vi "main_Extended-Kalman Filter.vi"() -> ()   [LabVIEW 2019]
uses:
  <vilib>/Analysis/Matrix/Datatypes/RealMatrix.ctl
  Ctrl/cmd_common.ctl
  Ctrl/cmd_ini-RW.ctl
  <vilib>/Analysis/Matrix/NI_Matrix.lvlib
panel:
  in  "tab":enum32{"ini val", "Graph"}(tab)=enum."Graph"
  out "GNSS Lat-Long":T1(graph)=[{[{"Real Matrix Element"=0.00648229933015812, "Real Matrix Element"=-0.1485998715838205}, {"Real Matrix Element"=0.13764030324676432, "Real Matrix Element"=-0.031872708572077454}, {"Real Matrix Element"=0.2814176053656353, "Real Matrix Element"=-0.18668844986322813}, {"Real Matrix Element"=0.4677656590914504, "Real Matrix Element"=-0.0031668042546943997}, {"Real Matrix Element"=0.4503900731423714, "Real Matrix Element"=-0.03691015780949122}, {"Real Matrix Element"=0.49534101114982676, "Real Matrix Element"=-0.0424373953622008}, {"Real Matrix Element"=0.5298272405394908, "Real Matrix Element"=-0.018737920527740447}, {"Real Matrix Element"=0.6136709918692839, "Real Matrix Element"=-0.07905311271886954}, {"Real Matrix Element"=0.8672293050090724, "Real Matrix Element"=0.11930935270810816}, {"Real Matrix Element"=1.032724976114411, "Real Matrix Element"=-0.028094767288573047}, {"Real Matrix Element"=1.025639298375923, "Real Matrix Element"=-0.015205341516983151}, {"Real Matrix Element"=1.0403214942691346, "Real Matrix Element"=0.10295017559703463}, {"Real Matrix Element"=1.2192703763694923, "Real Matrix Element"=0.2632396677335336}, {"Real Matrix Element"=1.2484932187390043, "Real Matrix Element"=0.11930141709508046}, {"Real Matrix Element"=1.28679874101843, "Real Matrix Element"=0.3188853450127311}, {"Real Matrix Element"=1.2528049501602503, "Real Matrix Element"=0.20840561524288012}, {"Real Matrix Element"=1.5260015333317185, "Real Matrix Element"=0.20710760450243698}, {"Real Matrix Element"=1.5664918211546404, "Real Matrix Element"=0.13271924379662997}, {"Real Matrix Element"=1.8460444096776403, "Real Matrix Element"=0.2388525674226506}, {"Real Matrix Element"=1.7893086393547315, "Real Matrix Element"=0.23473315440221695}, {"Real Matrix Element"=2.1003619347831006, "Real Matrix Element"=0.18965751247444596}, {"Real Matrix Element"=2.1527235912017235, "Real Matrix Element"=0.21292351546767185}, {"Real Matrix Element"=2.0471398164787855, "Real Matrix Element"=0.24502152593798443}, {"Real Matrix Element"=2.246363828219961, "Real Matrix Element"=0.21555940024166098}, {"Real Matrix Element"=2.3610927477240558, "Real Matrix Element"=0.2478574057445659}, {"Real Matrix Element"=2.4439556028948055, "Real Matrix Element"=0.34991078944230897}, {"Real Matrix Element"=2.4855190346914235, "Real Matrix Element"=0.4958049830178777}, {"Real Matrix Element"=2.677137946482532, "Real Matrix Element"=0.415459813566203}, {"Real Matrix Element"=2.8400473959196373, "Real Matrix Element"=0.3729959888015044}, {"Real Matrix Element"=2.8126782352199013, "Real Matrix Element"=0.3900898497303645}, {"Real Matrix Element"=3.0316200287530095, "Real Matrix Element"=0.41711101629898045}, {"Real Matrix Element"=3.159342773172584, "Real Matrix Element"=0.48895603096833595}, {"Real Matrix Element"=3.1177640465501595, "Real Matrix Element"=0.5990497173429132}, {"Real Matrix Element"=3.431510484521816, "Real Matrix Element"=0.6923490256189043}, {"Real Matrix Element"=3.6265865881623625, "Real Matrix Element"=0.7358839573835992}, {"Real Matrix Element"=3.678232807948232, "Real Matrix Element"=0.68180069643571}, {"Real Matrix Element"=3.765659578050578, "Real Matrix Element"=0.8018945377182328}, {"Real Matrix Element"=3.6248552222086228, "Real Matrix Element"=0.4741738414926855}, {"Real Matrix Element"=3.7222020295046874, "Real Matrix Element"=0.518341799011495}, {"Real Matrix Element"=3.9502494355664957, "Real Matrix Element"=0.7844506067834873}, {"Real Matrix Element"=4.140443942092801, "Real Matrix Element"=0.6861077494054908}, {"Real Matrix Element"=4.329408585769923, "Real Matrix Element"=0.9587932783737416}, {"Real Matrix Element"=4.4518189256360055, "Real Matrix Element"=0.9438312142162951}, {"Real Matrix Element"=4.565733385367433, "Real Matrix Element"=0.9829122817561525}, {"Real Matrix Element"=4.6100291786353536, "Real Matrix Element"=1.0160060370690478}, {"Real Matrix Element"=4.682015899254993, "Real Matrix Element"=1.1774809714765537}, {"Real Matrix Element"=4.732474262362473, "Real Matrix Element"=1.2571329943283698}, {"Real Matrix Element"=4.6216704645451285, "Real Matrix Element"=0.7679884807807758}, {"Real Matrix Element"=4.794245939393425, "Real Matrix Element"=0.7679902776857672}, {"Real Matrix Element"=4.856828698615568, "Real Matrix Element"=0.8294593794196793}, {"Real Matrix Element"=5.006091376727372, "Real Matrix Element"=0.9850119127052693}, {"Real Matrix Element"=5.173313411136047, "Real Matrix Element"=1.291609237984442}, {"Real Matrix Element"=5.196884811093232, "Real Matrix Element"=1.438539845070721}, {"Real Matrix Element"=5.269297502943308, "Real Matrix Element"=1.3591797613509908}, {"Real Matrix Element"=5.326632454975217, "Real Matrix Element"=1.5019081952917732}, {"Real Matrix Element"=5.53950476112955, "Real Matrix Element"=1.5954667192482002}, {"Real Matrix Element"=5.546075834353704, "Real Matrix Element"=1.5963373800411635}, {"Real Matrix Element"=5.50787264268229, "Real Matrix Element"=1.5136014331108896}, {"Real Matrix Element"=5.597318829657093, "Real Matrix Element"=1.6911722909521052}, {"Real Matrix Element"=5.745469013544655, "Real Matrix Element"=1.9741214083072083}, {"Real Matrix Element"=5.826534676656871, "Real Matrix Element"=1.8362557577429413}, {"Real Matrix Element"=5.777420682360288, "Real Matrix Element"=1.6471604684917265}, {"Real Matrix Element"=5.783642698159415, "Real Matrix Element"=1.7983117212024493}, {"Real Matrix Element"=5.77706746416779, "Real Matrix Element"=1.5876776162294384}, {"Real Matrix Element"=6.070669468161333, "Real Matrix Element"=2.0406137236959054}, {"Real Matrix Element"=6.1820279880490645, "Real Matrix Element"=2.043202141200636}, {"Real Matrix Element"=6.219822211005529, "Real Matrix Element"=2.099773718842126}, {"Real Matrix Element"=6.295561619993403, "Real Matrix Element"=1.9409629598593416}, {"Real Matrix Element"=6.439200544048959, "Real Matrix Element"=2.0875731372661637}, {"Real Matrix Element"=6.457028372016953, "Real Matrix Element"=2.203865379008531}, {"Real Matrix Element"=6.4704852502079975, "Real Matrix Element"=2.6003188639731913}, {"Real Matrix Element"=6.554666254302385, "Real Matrix Element"=2.503194424454099}, {"Real Matrix Element"=6.5733554844620565, "Real Matrix Element"=2.480092898008009}, {"Real Matrix Element"=6.754152844278384, "Real Matrix Element"=2.728791386153097}, {"Real Matrix Element"=6.674564513462208, "Real Matrix Element"=2.300939933732716}, {"Real Matrix Element"=6.691289619645367, "Real Matrix Element"=2.559983090203076}, {"Real Matrix Element"=6.8947220042735005, "Real Matrix Element"=2.7230740025712734}, {"Real Matrix Element"=7.015805006692874, "Real Matrix Element"=2.9921120011808027}, {"Real Matrix Element"=7.134483557016957, "Real Matrix Element"=2.887264461377884}, {"Real Matrix Element"=7.102799773965878, "Real Matrix Element"=2.863049574205883}, {"Real Matrix Element"=7.096532109525193, "Real Matrix Element"=3.000878596933252}, {"Real Matrix Element"=7.278203294615071, "Real Matrix Element"=3.2591886274505706}, {"Real Matrix Element"=7.267274013305502, "Real Matrix Element"=3.239806978191403}, {"Real Matrix Element"=7.432382425022456, "Real Matrix Element"=3.5891598453443536}, {"Real Matrix Element"=7.412170502397272, "Real Matrix Element"=3.4593252300230164}, {"Real Matrix Element"=7.535515352097216, "Real Matrix Element"=3.550645213044657}, {"Real Matrix Element"=7.735555416947001, "Real Matrix Element"=3.6444852552704137}, {"Real Matrix Element"=7.792479661433866, "Real Matrix Element"=3.5591098996316397}, {"Real Matrix Element"=7.932826704204354, "Real Matrix Element"=3.895277482405934}, {"Real Matrix Element"=7.873200422033903, "Real Matrix Element"=3.643453113387131}, {"Real Matrix Element"=7.9872990985151935, "Real Matrix Element"=3.7482458583440232}, {"Real Matrix Element"=8.023783453842626, "Real Matrix Element"=3.908963545529375}, {"Real Matrix Element"=8.090971345781176, "Real Matrix Element"=4.158683909791595}, {"Real Matrix Element"=8.179024885407793, "Real Matrix Element"=4.396388435221577}, {"Real Matrix Element"=8.244443630526025, "Real Matrix Element"=4.5010787950401925}, {"Real Matrix Element"=8.175467225219704, "Real Matrix Element"=4.304323569685333}, {"Real Matrix Element"=8.192177808998313, "Real Matrix Element"=4.296358269859259}, {"Real Matrix Element"=8.264968809143058, "Real Matrix Element"=4.25581006734387}, {"Real Matrix Element"=8.36355332414695, "Real Matrix Element"=4.410547430378274}, {"Real Matrix Element"=8.418999830088936, "Real Matrix Element"=4.441577526445436}, {"Real Matrix Element"=8.562267588591794, "Real Matrix Element"=4.527930122835036}, {"Real Matrix Element"=8.520294036398598, "Real Matrix Element"=4.864102834164672}, {"Real Matrix Element"=8.636696088427488, "Real Matrix Element"=4.9782078037972}, {"Real Matrix Element"=8.713850366189384, "Real Matrix Element"=4.962690664747354}, {"Real Matrix Element"=8.764321844517646, "Real Matrix Element"=5.114081495990158}, {"Real Matrix Element"=8.847549669446503, "Real Matrix Element"=5.218346627649721}, {"Real Matrix Element"=8.827369626773182, "Real Matrix Element"=5.021489079132804}, {"Real Matrix Element"=8.903059713218287, "Real Matrix Element"=5.235767123116211}, {"Real Matrix Element"=8.963155178977614, "Real Matrix Element"=5.598077779344656}, {"Real Matrix Element"=8.987948084499166, "Real Matrix Element"=5.597411139757482}, {"Real Matrix Element"=8.968808580972492, "Real Matrix Element"=5.645722006826326}, {"Real Matrix Element"=9.113001823113587, "Real Matrix Element"=5.60411213366905}, {"Real Matrix Element"=9.173522281833215, "Real Matrix Element"=5.852524519544907}, {"Real Matrix Element"=9.17913802407535, "Real Matrix Element"=6.032383124796971}, {"Real Matrix Element"=9.232914231961534, "Real Matrix Element"=5.837227051561382}, {"Real Matrix Element"=9.32071271816769, "Real Matrix Element"=6.001382731775994}, {"Real Matrix Element"=9.432490446545314, "Real Matrix Element"=6.077384745280501}, {"Real Matrix Element"=9.599670577348716, "Real Matrix Element"=6.3096112031527944}, {"Real Matrix Element"=9.671538974157912, "Real Matrix Element"=6.273083960801199}, {"Real Matrix Element"=9.577958664052026, "Real Matrix Element"=6.2972763478809926}, {"Real Matrix Element"=9.62603714326331, "Real Matrix Element"=6.374956836079589}, {"Real Matrix Element"=9.835344466832757, "Real Matrix Element"=6.4637793043762946}, {"Real Matrix Element"=9.909203846785434, "Real Matrix Element"=6.872950958027769}, {"Real Matrix Element"=9.840759582646996, "Real Matrix Element"=6.722130787954949}, {"Real Matrix Element"=9.973720776756435, "Real Matrix Element"=6.985178872427905}, {"Real Matrix Element"=9.945020881597433, "Real Matrix Element"=7.0799896615141265}, {"Real Matrix Element"=10.019541195927266, "Real Matrix Element"=6.961037799237819}, {"Real Matrix Element"=10.029458760055693, "Real Matrix Element"=6.770951391743203}, {"Real Matrix Element"=9.95680039378121, "Real Matrix Element"=6.894932057458966}, {"Real Matrix Element"=9.972679986203673, "Real Matrix Element"=7.097027209828476}, {"Real Matrix Element"=10.068459547490654, "Real Matrix Element"=7.346327751875404}, {"Real Matrix Element"=10.151213352812169, "Real Matrix Element"=7.3336762919149505}, {"Real Matrix Element"=10.090891521075756, "Real Matrix Element"=7.530166753288197}, {"Real Matrix Element"=10.147224053917913, "Real Matrix Element"=7.8719545623908855}, {"Real Matrix Element"=10.247445130984264, "Real Matrix Element"=8.059616854073887}, {"Real Matrix Element"=10.29353595886074, "Real Matrix Element"=7.9879086674452715}, {"Real Matrix Element"=10.226581274584332, "Real Matrix Element"=8.14872711101871}, {"Real Matrix Element"=10.182657003096221, "Real Matrix Element"=7.979886222894717}, {"Real Matrix Element"=10.170170736983122, "Real Matrix Element"=8.210361178998122}, {"Real Matrix Element"=10.221301770259442, "Real Matrix Element"=8.19710414327885}, {"Real Matrix Element"=10.23122536653524, "Real Matrix Element"=8.41557432626885}, {"Real Matrix Element"=10.22909019102822, "Real Matrix Element"=8.295293137067564}, {"Real Matrix Element"=10.36739039274229, "Real Matrix Element"=8.445827694791747}, {"Real Matrix Element"=10.39450178371217, "Real Matrix Element"=8.704741369116837}, {"Real Matrix Element"=10.568638625081983, "Real Matrix Element"=8.846568127767178}, {"Real Matrix Element"=10.559977944425762, "Real Matrix Element"=8.876524284264356}, {"Real Matrix Element"=10.696128835374578, "Real Matrix Element"=8.909886242456711}, {"Real Matrix Element"=10.68613966102341, "Real Matrix Element"=9.225666737988437}, {"Real Matrix Element"=10.638910101463535, "Real Matrix Element"=9.200847051506699}, {"Real Matrix Element"=10.641981226688847, "Real Matrix Element"=9.228452429971046}, {"Real Matrix Element"=10.65517617340279, "Real Matrix Element"=9.220194949369594}, {"Real Matrix Element"=10.691934312144625, "Real Matrix Element"=9.220574387761589}, {"Real Matrix Element"=10.856493342491829, "Real Matrix Element"=9.456143755756003}, {"Real Matrix Element"=10.748481161304678, "Real Matrix Element"=9.660792312776644}, {"Real Matrix Element"=10.730109086692375, "Real Matrix Element"=9.661757950863059}, {"Real Matrix Element"=10.71249938490896, "Real Matrix Element"=9.88205892199337}, {"Real Matrix Element"=10.519708404690254, "Real Matrix Element"=9.633758525080326}, {"Real Matrix Element"=10.537028139820096, "Real Matrix Element"=9.711517025179154}, {"Real Matrix Element"=10.611910728524084, "Real Matrix Element"=9.846185660821696}, {"Real Matrix Element"=10.651966971953641, "Real Matrix Element"=9.956538412771572}, {"Real Matrix Element"=10.716055814283216, "Real Matrix Element"=10.181348255220488}, {"Real Matrix Element"=10.738690953168351, "Real Matrix Element"=10.195158981215268}, {"Real Matrix Element"=10.81569244536906, "Real Matrix Element"=10.333686183942001}, {"Real Matrix Element"=10.891289126354476, "Real Matrix Element"=10.647008375840068}, {"Real Matrix Element"=10.945229634349461, "Real Matrix Element"=10.356736595320573}, {"Real Matrix Element"=11.036714501214382, "Real Matrix Element"=10.433679401177264}, {"Real Matrix Element"=11.095978460860579, "Real Matrix Element"=10.834554613260545}, {"Real Matrix Element"=10.962880721495313, "Real Matrix Element"=10.721611576289368}, {"Real Matrix Element"=10.945970437104213, "Real Matrix Element"=10.777251776751498}, {"Real Matrix Element"=10.858418050644882, "Real Matrix Element"=11.106073137748869}, {"Real Matrix Element"=10.992624941935272, "Real Matrix Element"=11.486243688704834}, {"Real Matrix Element"=10.738788257878593, "Real Matrix Element"=10.956412747643766}, {"Real Matrix Element"=10.883062812427877, "Real Matrix Element"=11.020596690664222}, {"Real Matrix Element"=11.107212545404389, "Real Matrix Element"=11.425304671954585}, {"Real Matrix Element"=11.067696675081926, "Real Matrix Element"=11.512956937565612}, {"Real Matrix Element"=11.160753482337359, "Real Matrix Element"=11.55748715945855}, {"Real Matrix Element"=11.073554637302253, "Real Matrix Element"=11.763495460705855}, {"Real Matrix Element"=11.138923802464973, "Real Matrix Element"=11.984706913691065}, {"Real Matrix Element"=11.155131070521213, "Real Matrix Element"=12.000895635212945}, {"Real Matrix Element"=11.156829831662023, "Real Matrix Element"=11.91719637666095}, {"Real Matrix Element"=11.135853359663102, "Real Matrix Element"=12.064860774008855}, {"Real Matrix Element"=11.0397135228759, "Real Matrix Element"=12.157997080156921}, {"Real Matrix Element"=11.104505632643955, "Real Matrix Element"=12.093158641244708}, {"Real Matrix Element"=11.032171697903264, "Real Matrix Element"=12.016222884836482}, {"Real Matrix Element"=11.014993286595812, "Real Matrix Element"=12.226762016183388}, {"Real Matrix Element"=11.030470414809848, "Real Matrix Element"=12.335822302519217}, {"Real Matrix Element"=10.744696405687874, "Real Matrix Element"=12.369922735789935}, {"Real Matrix Element"=10.563658451027987, "Real Matrix Element"=12.342965988768649}, {"Real Matrix Element"=10.558977903584646, "Real Matrix Element"=12.420112129106617}, {"Real Matrix Element"=10.689454055342747, "Real Matrix Element"=12.629368569941006}, {"Real Matrix Element"=10.850725649755843, "Real Matrix Element"=12.690142184061555}, {"Real Matrix Element"=10.859890034332354, "Real Matrix Element"=12.88044758109158}, {"Real Matrix Element"=10.902675181913143, "Real Matrix Element"=13.11104319804944}, {"Real Matrix Element"=10.773398062223649, "Real Matrix Element"=13.083576841459834}, {"Real Matrix Element"=10.689147628816622, "Real Matrix Element"=12.982525656460956}, {"Real Matrix Element"=10.73177241965574, "Real Matrix Element"=13.284545355525509}, {"Real Matrix Element"=10.636957344960486, "Real Matrix Element"=13.32885598676617}, {"Real Matrix Element"=10.47701460100469, "Real Matrix Element"=13.470653974564684}, {"Real Matrix Element"=10.611979714767, "Real Matrix Element"=13.614521334694713}, {"Real Matrix Element"=10.667772132564563, "Real Matrix Element"=13.815801586008588}, {"Real Matrix Element"=10.572778256295816, "Real Matrix Element"=13.66197393739574}, {"Real Matrix Element"=10.547381882820277, "Real Matrix Element"=13.873879718186835}, {"Real Matrix Element"=10.497919032969687, "Real Matrix Element"=13.93962191703575}, {"Real Matrix Element"=10.441409465937898, "Real Matrix Element"=14.069828248852192}, {"Real Matrix Element"=10.416888740730123, "Real Matrix Element"=14.281262804810398}, {"Real Matrix Element"=10.365853199762403, "Real Matrix Element"=14.319036535656323}, {"Real Matrix Element"=10.382347444727786, "Real Matrix Element"=14.494998192788628}, {"Real Matrix Element"=10.3412155257497, "Real Matrix Element"=14.486270865832722}, {"Real Matrix Element"=10.159664187026435, "Real Matrix Element"=14.53549207632453}, {"Real Matrix Element"=10.196640847527227, "Real Matrix Element"=14.800251855397082}, {"Real Matrix Element"=10.098370928407073, "Real Matrix Element"=14.74592086075482}, {"Real Matrix Element"=10.061317266994362, "Real Matrix Element"=14.894832915663956}, {"Real Matrix Element"=10.117914758481051, "Real Matrix Element"=15.076274138651362}, {"Real Matrix Element"=10.033154142179235, "Real Matrix Element"=15.079952353641815}, {"Real Matrix Element"=10.05100120761777, "Real Matrix Element"=15.077175387635783}, {"Real Matrix Element"=9.961391196845407, "Real Matrix Element"=14.918803681368212}, {"Real Matrix Element"=9.840461007257934, "Real Matrix Element"=15.010931484147449}, {"Real Matrix Element"=9.822982863269367, "Real Matrix Element"=15.122339825609382}, {"Real Matrix Element"=9.728412122409905, "Real Matrix Element"=15.167624367981539}, {"Real Matrix Element"=9.769321903635342, "Real Matrix Element"=15.42312836015468}, {"Real Matrix Element"=9.705347680257447, "Real Matrix Element"=15.24533840587037}, {"Real Matrix Element"=9.572140055944566, "Real Matrix Element"=15.26307722189673}, {"Real Matrix Element"=9.626449698046892, "Real Matrix Element"=15.451020045895378}, {"Real Matrix Element"=9.563687615025065, "Real Matrix Element"=15.447593898483193}, {"Real Matrix Element"=9.477196367990114, "Real Matrix Element"=15.289000648370846}, {"Real Matrix Element"=9.508922089175302, "Real Matrix Element"=15.632120856342432}, {"Real Matrix Element"=9.308497528813842, "Real Matrix Element"=15.702924505578798}, {"Real Matrix Element"=9.210428787966308, "Real Matrix Element"=15.752032751967723}, {"Real Matrix Element"=9.255548728935418, "Real Matrix Element"=15.855908881085199}, {"Real Matrix Element"=9.257040936226382, "Real Matrix Element"=15.972723917928441}, {"Real Matrix Element"=9.210793751209403, "Real Matrix Element"=16.20154327768208}, {"Real Matrix Element"=9.14745231932969, "Real Matrix Element"=16.34668846312586}, {"Real Matrix Element"=9.060419639163928, "Real Matrix Element"=16.366748863943407}, {"Real Matrix Element"=9.109408723968903, "Real Matrix Element"=16.50727644323798}, {"Real Matrix Element"=9.019710189144376, "Real Matrix Element"=16.28433943957462}, {"Real Matrix Element"=8.940542818972272, "Real Matrix Element"=16.47647079065354}, {"Real Matrix Element"=8.942496897635841, "Real Matrix Element"=16.542827768454348}, {"Real Matrix Element"=8.813052139267528, "Real Matrix Element"=16.719265379563524}, {"Real Matrix Element"=8.71449519310659, "Real Matrix Element"=16.697936477297915}, {"Real Matrix Element"=8.58276913696831, "Real Matrix Element"=16.749144759759258}, {"Real Matrix Element"=8.42811254248165, "Real Matrix Element"=16.830853513545733}, {"Real Matrix Element"=8.3352788450772, "Real Matrix Element"=16.867495644823915}, {"Real Matrix Element"=8.012518887672181, "Real Matrix Element"=16.641065468893878}, {"Real Matrix Element"=8.01825470695931, "Real Matrix Element"=16.780837214405047}, {"Real Matrix Element"=7.899234473922093, "Real Matrix Element"=16.993908720759837}, {"Real Matrix Element"=7.7939150629363905, "Real Matrix Element"=17.15981951856707}, {"Real Matrix Element"=7.642718395610258, "Real Matrix Element"=17.333737224286455}, {"Real Matrix Element"=7.593601714301942, "Real Matrix Element"=17.63394458542353}, {"Real Matrix Element"=7.458544359951948, "Real Matrix Element"=17.525938480144106}, {"Real Matrix Element"=7.446227547565758, "Real Matrix Element"=17.61485439269415}, {"Real Matrix Element"=7.4267155874547335, "Real Matrix Element"=17.8069966855528}, {"Real Matrix Element"=7.297223883018756, "Real Matrix Element"=17.7765035138789}, {"Real Matrix Element"=7.2176263326083525, "Real Matrix Element"=17.68979842828898}, {"Real Matrix Element"=7.107712135235226, "Real Matrix Element"=17.88435508692095}, {"Real Matrix Element"=6.98865643585801, "Real Matrix Element"=18.12296772431429}, {"Real Matrix Element"=6.903000301233418, "Real Matrix Element"=17.953595941493052}, {"Real Matrix Element"=6.953305506197489, "Real Matrix Element"=17.88066771121086}, {"Real Matrix Element"=6.964430081263262, "Real Matrix Element"=18.29539097213008}, {"Real Matrix Element"=6.886151514415655, "Real Matrix Element"=18.195631674332745}, {"Real Matrix Element"=6.7336229763437645, "Real Matrix Element"=18.132614920947365}, {"Real Matrix Element"=6.59529073795722, "Real Matrix Element"=18.129690386956742}, {"Real Matrix Element"=6.421457979860058, "Real Matrix Element"=18.097688814401582}, {"Real Matrix Element"=6.313687471615972, "Real Matrix Element"=18.256075347070862}, {"Real Matrix Element"=6.424693836858833, "Real Matrix Element"=18.385104065732463}, {"Real Matrix Element"=6.314037480333121, "Real Matrix Element"=18.48053996622295}, {"Real Matrix Element"=6.282274976322439, "Real Matrix Element"=18.474245114045907}, {"Real Matrix Element"=6.17859079036297, "Real Matrix Element"=18.364168550574856}, {"Real Matrix Element"=6.028222503746511, "Real Matrix Element"=18.343099331132105}, {"Real Matrix Element"=6.041830014182925, "Real Matrix Element"=18.734058842793605}, {"Real Matrix Element"=5.817884322878366, "Real Matrix Element"=18.729095853732442}, {"Real Matrix Element"=5.728528409685127, "Real Matrix Element"=18.423985690764976}, {"Real Matrix Element"=5.737897915893743, "Real Matrix Element"=18.497673467636595}, {"Real Matrix Element"=5.88089573337273, "Real Matrix Element"=18.875753032647165}, {"Real Matrix Element"=5.799770228009964, "Real Matrix Element"=19.175195922333323}, {"Real Matrix Element"=5.789559971988034, "Real Matrix Element"=19.14148484617277}, {"Real Matrix Element"=5.728620529283469, "Real Matrix Element"=19.03955848908346}, {"Real Matrix Element"=5.610959473946475, "Real Matrix Element"=19.01126576064702}, {"Real Matrix Element"=5.468725930097043, "Real Matrix Element"=18.95934887507015}, {"Real Matrix Element"=5.258312392053178, "Real Matrix Element"=18.84099422883017}, {"Real Matrix Element"=5.142446342313342, "Real Matrix Element"=18.90305594213509}, {"Real Matrix Element"=5.105882999072948, "Real Matrix Element"=19.083918286623355}, {"Real Matrix Element"=4.969139221496077, "Real Matrix Element"=19.0712670542347}, {"Real Matrix Element"=4.88310518463363, "Real Matrix Element"=18.991517734004915}, {"Real Matrix Element"=4.883449745637362, "Real Matrix Element"=19.23764693208351}, {"Real Matrix Element"=4.858716495531576, "Real Matrix Element"=19.23079595747254}, {"Real Matrix Element"=4.553529904374067, "Real Matrix Element"=19.07229252484832}, {"Real Matrix Element"=4.349863782646297, "Real Matrix Element"=19.037674133821874}, {"Real Matrix Element"=4.293894605322258, "Real Matrix Element"=19.13986289418251}, {"Real Matrix Element"=4.216049493928996, "Real Matrix Element"=19.17121274363941}, {"Real Matrix Element"=4.161383022443987, "Real Matrix Element"=19.191447872463566}, {"Real Matrix Element"=4.0530417215637025, "Real Matrix Element"=19.186800211457566}, {"Real Matrix Element"=4.042648839031042, "Real Matrix Element"=19.15859018809776}, {"Real Matrix Element"=3.8708313571383637, "Real Matrix Element"=18.98630569595587}, {"Real Matrix Element"=3.7861624113717705, "Real Matrix Element"=19.02282756929192}, {"Real Matrix Element"=3.6248212985013524, "Real Matrix Element"=19.0542132473345}, {"Real Matrix Element"=3.5398824631699077, "Real Matrix Element"=19.23663553943419}, {"Real Matrix Element"=3.518418289613293, "Real Matrix Element"=19.376029715074676}, {"Real Matrix Element"=3.5463386912910444, "Real Matrix Element"=19.473742296659434}, {"Real Matrix Element"=3.377113972824625, "Real Matrix Element"=19.510879952760902}, {"Real Matrix Element"=3.157897228180288, "Real Matrix Element"=19.487434858471588}, {"Real Matrix Element"=2.9436884312738893, "Real Matrix Element"=19.42809192809007}, {"Real Matrix Element"=2.838590666851104, "Real Matrix Element"=19.29426924054106}, {"Real Matrix Element"=2.857927587538658, "Real Matrix Element"=19.556715271253456}, {"Real Matrix Element"=2.814896864898186, "Real Matrix Element"=19.717000998204135}, {"Real Matrix Element"=2.6408949188102757, "Real Matrix Element"=19.643173344483763}, {"Real Matrix Element"=2.541876363101788, "Real Matrix Element"=19.67189648166023}, {"Real Matrix Element"=2.398493755855199, "Real Matrix Element"=19.716988032260204}, {"Real Matrix Element"=2.2527560041587007, "Real Matrix Element"=19.77217050768258}, {"Real Matrix Element"=2.2385637434975085, "Real Matrix Element"=19.804926414433083}, {"Real Matrix Element"=2.032480520028906, "Real Matrix Element"=19.70599721639635}, {"Real Matrix Element"=1.9251366567763575, "Real Matrix Element"=19.638292298885922}, {"Real Matrix Element"=1.8506901894879193, "Real Matrix Element"=19.689642573643777}, {"Real Matrix Element"=1.773609920595391, "Real Matrix Element"=19.74291251685918}, {"Real Matrix Element"=1.8129589817161393, "Real Matrix Element"=19.62285094891314}, {"Real Matrix Element"=1.7839150038940164, "Real Matrix Element"=19.579173511245667}, {"Real Matrix Element"=1.6715193986570722, "Real Matrix Element"=19.66520025814235}, {"Real Matrix Element"=1.563721984487164, "Real Matrix Element"=19.83849159438622}, {"Real Matrix Element"=1.4979890477860904, "Real Matrix Element"=19.665613829119632}, {"Real Matrix Element"=1.2903941207181793, "Real Matrix Element"=19.458592458591937}, {"Real Matrix Element"=1.179428589652568, "Real Matrix Element"=19.5696145212218}, {"Real Matrix Element"=1.0632572185390148, "Real Matrix Element"=19.813823164962702}, {"Real Matrix Element"=1.1061520183981444, "Real Matrix Element"=19.59766246002792}, {"Real Matrix Element"=1.1242462783354095, "Real Matrix Element"=19.56317950186761}, {"Real Matrix Element"=1.0593901157736048, "Real Matrix Element"=19.596015963603698}, {"Real Matrix Element"=0.9030850669069698, "Real Matrix Element"=19.313662268429287}, {"Real Matrix Element"=0.7123477149575078, "Real Matrix Element"=19.38568414958826}, {"Real Matrix Element"=0.6252156697315172, "Real Matrix Element"=19.423829204687465}, {"Real Matrix Element"=0.46667037481651064, "Real Matrix Element"=19.50778350974887}, {"Real Matrix Element"=0.300414478688687, "Real Matrix Element"=19.549185575108226}, {"Real Matrix Element"=0.09691991033420871, "Real Matrix Element"=19.39960382837237}, {"Real Matrix Element"=-0.212128689581318, "Real Matrix Element"=19.274595827567577}, {"Real Matrix Element"=-0.2445828930637551, "Real Matrix Element"=19.31812900551943}, {"Real Matrix Element"=-0.4463995472266077, "Real Matrix Element"=19.18217998887929}, {"Real Matrix Element"=-0.5668976779085617, "Real Matrix Element"=19.164632720217423}, {"Real Matrix Element"=-0.6797563881516864, "Real Matrix Element"=19.381118353413477}, {"Real Matrix Element"=-0.5913170913339922, "Real Matrix Element"=19.64494016125629}, {"Real Matrix Element"=-0.8093517101665189, "Real Matrix Element"=19.435151434916417}, {"Real Matrix Element"=-0.9113181305923131, "Real Matrix Element"=19.469298865244877}, {"Real Matrix Element"=-0.9618035892484105, "Real Matrix Element"=19.54373992583285}, {"Real Matrix Element"=-1.2055803280850832, "Real Matrix Element"=19.508843606786723}, {"Real Matrix Element"=-1.074125842764567, "Real Matrix Element"=19.508384155795063}, {"Real Matrix Element"=-1.2000672089750195, "Real Matrix Element"=19.4252499391578}, {"Real Matrix Element"=-1.3220461408787072, "Real Matrix Element"=19.112338548032003}, {"Real Matrix Element"=-1.4716382582838243, "Real Matrix Element"=19.094029900238365}, {"Real Matrix Element"=-1.5112711250262618, "Real Matrix Element"=19.166501812121304}, {"Real Matrix Element"=-1.813648221913847, "Real Matrix Element"=18.907741535657028}, {"Real Matrix Element"=-1.9996265486940057, "Real Matrix Element"=18.909215446662262}, {"Real Matrix Element"=-2.0443919716231793, "Real Matrix Element"=19.026906661300956}, {"Real Matrix Element"=-2.2246729892602404, "Real Matrix Element"=19.1982995377807}, {"Real Matrix Element"=-2.310166519779252, "Real Matrix Element"=19.149554635045057}, {"Real Matrix Element"=-2.403059089215609, "Real Matrix Element"=19.140260311189053}, {"Real Matrix Element"=-2.514230275062345, "Real Matrix Element"=19.05415044998753}, {"Real Matrix Element"=-2.6974238146595373, "Real Matrix Element"=18.925614136937252}, {"Real Matrix Element"=-2.663083235121508, "Real Matrix Element"=18.989614949381398}, {"Real Matrix Element"=-2.8666200904088845, "Real Matrix Element"=18.908053440625746}, {"Real Matrix Element"=-2.8692981405928735, "Real Matrix Element"=19.030630558919018}, {"Real Matrix Element"=-2.930870024021501, "Real Matrix Element"=19.050038852489774}, {"Real Matrix Element"=-3.006249937553372, "Real Matrix Element"=18.894784085576326}, {"Real Matrix Element"=-3.1056563600967713, "Real Matrix Element"=18.71907527980109}, {"Real Matrix Element"=-3.2525410013236327, "Real Matrix Element"=18.626190509194075}, {"Real Matrix Element"=-3.4203247104737757, "Real Matrix Element"=18.432786241910286}, {"Real Matrix Element"=-3.2966944935483733, "Real Matrix Element"=18.665334244846736}, {"Real Matrix Element"=-3.328321683844109, "Real Matrix Element"=18.46352980009375}, {"Real Matrix Element"=-3.465022105044825, "Real Matrix Element"=18.30762640695359}, {"Real Matrix Element"=-3.4941286118894466, "Real Matrix Element"=18.35089715761776}, {"Real Matrix Element"=-3.4570968847660017, "Real Matrix Element"=18.30801482242164}, {"Real Matrix Element"=-3.563680046686781, "Real Matrix Element"=18.509007756145525}, {"Real Matrix Element"=-3.668734847581237, "Real Matrix Element"=18.50836024501096}, {"Real Matrix Element"=-3.7970598337868737, "Real Matrix Element"=18.252224338246542}, {"Real Matrix Element"=-3.969449400014437, "Real Matrix Element"=18.276599443426996}, {"Real Matrix Element"=-4.123656879512641, "Real Matrix Element"=18.290033883198433}, {"Real Matrix Element"=-4.174642915449263, "Real Matrix Element"=18.308441019274394}, {"Real Matrix Element"=-3.9921562943324074, "Real Matrix Element"=18.506962096806692}, {"Real Matrix Element"=-4.138513836385282, "Real Matrix Element"=18.138151737374667}, {"Real Matrix Element"=-3.9922444198867986, "Real Matrix Element"=18.272277020476388}, {"Real Matrix Element"=-4.122420721423742, "Real Matrix Element"=17.966412258123643}, {"Real Matrix Element"=-4.107373902038159, "Real Matrix Element"=18.047659169631512}, {"Real Matrix Element"=-4.41768884214291, "Real Matrix Element"=17.747483307674617}, {"Real Matrix Element"=-4.441621878599124, "Real Matrix Element"=17.81104400271665}, {"Real Matrix Element"=-4.527381301278483, "Real Matrix Element"=17.58632583124384}, {"Real Matrix Element"=-4.607759158875099, "Real Matrix Element"=17.60286399373877}, {"Real Matrix Element"=-4.738530269816759, "Real Matrix Element"=17.569212996342223}, {"Real Matrix Element"=-4.844291364139435, "Real Matrix Element"=17.419087384310693}, {"Real Matrix Element"=-4.914812116820954, "Real Matrix Element"=17.48718150238326}, {"Real Matrix Element"=-5.0689457411916194, "Real Matrix Element"=17.395522729393043}, {"Real Matrix Element"=-5.102346974163554, "Real Matrix Element"=17.293398194519334}, {"Real Matrix Element"=-5.172722711570282, "Real Matrix Element"=17.303055301305104}, {"Real Matrix Element"=-5.366853968339292, "Real Matrix Element"=16.805701067838235}, {"Real Matrix Element"=-5.37580540846757, "Real Matrix Element"=16.91551965726558}, {"Real Matrix Element"=-5.523338016670559, "Real Matrix Element"=16.81750087443277}, {"Real Matrix Element"=-5.689095308817158, "Real Matrix Element"=17.0343315047758}, {"Real Matrix Element"=-5.84258939181878, "Real Matrix Element"=16.840885853548986}, {"Real Matrix Element"=-5.921947076219957, "Real Matrix Element"=16.72880006917487}, {"Real Matrix Element"=-6.000284801976608, "Real Matrix Element"=16.81442580951811}, {"Real Matrix Element"=-6.16702704514055, "Real Matrix Element"=16.58347758297331}, {"Real Matrix Element"=-6.263879069967023, "Real Matrix Element"=16.528416639827725}, {"Real Matrix Element"=-6.295467398941262, "Real Matrix Element"=16.43391964679536}, {"Real Matrix Element"=-6.3704005460702815, "Real Matrix Element"=16.56266860070164}, {"Real Matrix Element"=-6.471640459565302, "Real Matrix Element"=16.339108200678293}, {"Real Matrix Element"=-6.686599373658382, "Real Matrix Element"=16.29822428830749}, {"Real Matrix Element"=-6.762176800965342, "Real Matrix Element"=16.260831209320358}, {"Real Matrix Element"=-6.644601975185713, "Real Matrix Element"=16.29083658398962}, {"Real Matrix Element"=-6.847756502741931, "Real Matrix Element"=15.929816182334598}, {"Real Matrix Element"=-6.751178876615401, "Real Matrix Element"=16.18932326061118}, {"Real Matrix Element"=-6.860396041654662, "Real Matrix Element"=15.955052393886879}, {"Real Matrix Element"=-7.005111320568655, "Real Matrix Element"=15.811734283654996}, {"Real Matrix Element"=-7.0299983106081525, "Real Matrix Element"=15.885480338863024}, {"Real Matrix Element"=-7.01828858124578, "Real Matrix Element"=15.790636571602592}, {"Real Matrix Element"=-7.152708077364718, "Real Matrix Element"=15.78829121311867}, {"Real Matrix Element"=-7.140044698193229, "Real Matrix Element"=15.521877098095974}, {"Real Matrix Element"=-7.063804999665451, "Real Matrix Element"=15.623407261413917}, {"Real Matrix Element"=-7.271912893932602, "Real Matrix Element"=15.525685713617099}, {"Real Matrix Element"=-7.284200960177758, "Real Matrix Element"=15.397501640782414}, {"Real Matrix Element"=-7.278135876243757, "Real Matrix Element"=15.524650337410009}, {"Real Matrix Element"=-7.324931448455408, "Real Matrix Element"=15.50452395177066}, {"Real Matrix Element"=-7.4411967229909175, "Real Matrix Element"=15.267055307626151}, {"Real Matrix Element"=-7.512597157378444, "Real Matrix Element"=15.03271788741639}, {"Real Matrix Element"=-7.709079548092833, "Real Matrix Element"=15.101616958024882}, {"Real Matrix Element"=-7.788613860068299, "Real Matrix Element"=15.028783742219797}, {"Real Matrix Element"=-7.708204674086434, "Real Matrix Element"=15.029379946850373}, {"Real Matrix Element"=-7.8375831184593965, "Real Matrix Element"=14.674922092285154}, {"Real Matrix Element"=-7.916646002532581, "Real Matrix Element"=14.762690905560362}, {"Real Matrix Element"=-7.921092911646018, "Real Matrix Element"=14.562554694780625}, {"Real Matrix Element"=-7.911069746602778, "Real Matrix Element"=14.497616380870802}, {"Real Matrix Element"=-7.924432800637839, "Real Matrix Element"=14.425217366935241}, {"Real Matrix Element"=-7.892270843693485, "Real Matrix Element"=14.27723738386671}, {"Real Matrix Element"=-7.892367939369549, "Real Matrix Element"=14.046063983104434}, {"Real Matrix Element"=-8.089353416004627, "Real Matrix Element"=13.93560323863065}, {"Real Matrix Element"=-8.244276415883338, "Real Matrix Element"=13.796414292109114}, {"Real Matrix Element"=-8.307806356072705, "Real Matrix Element"=13.82499256416825}, {"Real Matrix Element"=-8.45535395146506, "Real Matrix Element"=13.70931285975319}, {"Real Matrix Element"=-8.242446105999134, "Real Matrix Element"=13.972802707618929}, {"Real Matrix Element"=-8.250949449624512, "Real Matrix Element"=14.02633893856531}, {"Real Matrix Element"=-8.100353949872485, "Real Matrix Element"=13.957466114319974}, {"Real Matrix Element"=-8.39984263932783, "Real Matrix Element"=13.571747222280736}, {"Real Matrix Element"=-8.431651054067164, "Real Matrix Element"=13.297024196935372}, {"Real Matrix Element"=-8.399348184292883, "Real Matrix Element"=13.28761706920469}, {"Real Matrix Element"=-8.4138295056989, "Real Matrix Element"=13.125179340806694}, {"Real Matrix Element"=-8.50068093085815, "Real Matrix Element"=13.194921188887106}, {"Real Matrix Element"=-8.507485613228468, "Real Matrix Element"=13.250267458234559}, {"Real Matrix Element"=-8.643149478044451, "Real Matrix Element"=13.000933717634142}, {"Real Matrix Element"=-8.82622805362611, "Real Matrix Element"=12.822777889831777}, {"Real Matrix Element"=-8.905068886596476, "Real Matrix Element"=12.52406231926748}, {"Real Matrix Element"=-8.769123576961587, "Real Matrix Element"=12.50801959102291}, {"Real Matrix Element"=-8.729182433528239, "Real Matrix Element"=12.641628502730914}, {"Real Matrix Element"=-9.052897102068012, "Real Matrix Element"=12.41865224190188}, {"Real Matrix Element"=-8.98331784358087, "Real Matrix Element"=12.334719787390831}, {"Real Matrix Element"=-9.004055097908743, "Real Matrix Element"=12.288406545731188}, {"Real Matrix Element"=-9.168688660006698, "Real Matrix Element"=12.0977776050486}, {"Real Matrix Element"=-9.137575953926248, "Real Matrix Element"=12.202503889553364}, {"Real Matrix Element"=-9.309042052315192, "Real Matrix Element"=12.0337279625558}, {"Real Matrix Element"=-9.208664375640977, "Real Matrix Element"=12.253368352596844}, {"Real Matrix Element"=-9.083538767315991, "Real Matrix Element"=12.12327907253897}, {"Real Matrix Element"=-9.069569690260339, "Real Matrix Element"=11.916114470572898}, {"Real Matrix Element"=-9.144682641675463, "Real Matrix Element"=11.798739198876541}, {"Real Matrix Element"=-9.094874402449362, "Real Matrix Element"=11.61111152737767}, {"Real Matrix Element"=-9.23883571113969, "Real Matrix Element"=11.535796101681845}, {"Real Matrix Element"=-9.298806009127244, "Real Matrix Element"=11.474026974670888}, {"Real Matrix Element"=-9.382113857695996, "Real Matrix Element"=11.27024669494284}, {"Real Matrix Element"=-9.586069831830285, "Real Matrix Element"=11.053309234066706}, {"Real Matrix Element"=-9.418606633081371, "Real Matrix Element"=11.003227479317676}, {"Real Matrix Element"=-9.516042795851693, "Real Matrix Element"=10.800806922714445}, {"Real Matrix Element"=-9.5653285560924, "Real Matrix Element"=10.511371205766904}, {"Real Matrix Element"=-9.54395792978633, "Real Matrix Element"=10.370174559892918}, {"Real Matrix Element"=-9.442828547870754, "Real Matrix Element"=10.381399521910787}, {"Real Matrix Element"=-9.350609220450888, "Real Matrix Element"=10.330985850589}, {"Real Matrix Element"=-9.342066914735135, "Real Matrix Element"=10.416156843460685}, {"Real Matrix Element"=-9.38853189237257, "Real Matrix Element"=10.078288083686129}, {"Real Matrix Element"=-9.389224832954527, "Real Matrix Element"=10.179020171813702}, {"Real Matrix Element"=-9.261047031646248, "Real Matrix Element"=10.234807537176792}, {"Real Matrix Element"=-9.226057391262257, "Real Matrix Element"=9.968685662457396}, {"Real Matrix Element"=-9.380786404634934, "Real Matrix Element"=9.470446832878485}, {"Real Matrix Element"=-9.293085957516675, "Real Matrix Element"=9.502239181797504}, {"Real Matrix Element"=-9.316689747860538, "Real Matrix Element"=9.631853840919593}, {"Real Matrix Element"=-9.34212001555966, "Real Matrix Element"=9.34257621010338}, {"Real Matrix Element"=-9.415133051188548, "Real Matrix Element"=9.434136395073317}, {"Real Matrix Element"=-9.505985531498801, "Real Matrix Element"=9.383480328616004}, {"Real Matrix Element"=-9.384725356048321, "Real Matrix Element"=9.644438462922052}, {"Real Matrix Element"=-9.378093339453057, "Real Matrix Element"=9.414586234680899}, {"Real Matrix Element"=-9.55768144088628, "Real Matrix Element"=9.089358496271746}, {"Real Matrix Element"=-9.484550845650611, "Real Matrix Element"=8.933515994616805}, {"Real Matrix Element"=-9.421645461118713, "Real Matrix Element"=8.974223277725828}, {"Real Matrix Element"=-9.404344030958514, "Real Matrix Element"=8.940816169678031}, {"Real Matrix Element"=-9.390467526061752, "Real Matrix Element"=8.822816043821307}, {"Real Matrix Element"=-9.400085645431245, "Real Matrix Element"=8.680744783307954}, {"Real Matrix Element"=-9.498462733318572, "Real Matrix Element"=8.534121597735398}, {"Real Matrix Element"=-9.346298057132104, "Real Matrix Element"=8.476371870885595}, {"Real Matrix Element"=-9.296593549202104, "Real Matrix Element"=8.509355076877814}, {"Real Matrix Element"=-9.404262387210196, "Real Matrix Element"=8.233369886633618}, {"Real Matrix Element"=-9.402908432152197, "Real Matrix Element"=8.35393141819312}, {"Real Matrix Element"=-9.46062498131566, "Real Matrix Element"=8.034243614338454}, {"Real Matrix Element"=-9.405909591392097, "Real Matrix Element"=8.250499425905867}, {"Real Matrix Element"=-9.364359211798288, "Real Matrix Element"=8.042860181332038}, {"Real Matrix Element"=-9.409263081609572, "Real Matrix Element"=7.724994865873486}, {"Real Matrix Element"=-9.449699409366191, "Real Matrix Element"=7.738184298283442}, {"Real Matrix Element"=-9.402673384155545, "Real Matrix Element"=7.638426610067694}, {"Real Matrix Element"=-9.316396194070588, "Real Matrix Element"=7.561701110752079}, {"Real Matrix Element"=-9.343995684462689, "Real Matrix Element"=7.595551593434095}, {"Real Matrix Element"=-9.36275537744109, "Real Matrix Element"=7.482423507376256}, {"Real Matrix Element"=-9.32199058648848, "Real Matrix Element"=7.3383204384136205}, {"Real Matrix Element"=-9.255636696293417, "Real Matrix Element"=7.120305441269133}, {"Real Matrix Element"=-9.33197492036367, "Real Matrix Element"=6.720262531940557}, {"Real Matrix Element"=-9.39843863227546, "Real Matrix Element"=7.028623687041532}, {"Real Matrix Element"=-9.314540364393029, "Real Matrix Element"=6.930930066504008}, {"Real Matrix Element"=-9.235384737947685, "Real Matrix Element"=6.981588565556719}, {"Real Matrix Element"=-9.182278524154318, "Real Matrix Element"=6.593437716921817}, {"Real Matrix Element"=-9.082542015199683, "Real Matrix Element"=6.350569507278284}, {"Real Matrix Element"=-8.876527239530855, "Real Matrix Element"=6.632510881213491}, {"Real Matrix Element"=-8.865111751363465, "Real Matrix Element"=6.483978725787635}, {"Real Matrix Element"=-8.855623696436252, "Real Matrix Element"=6.136995349063769}, {"Real Matrix Element"=-8.848494770341604, "Real Matrix Element"=6.037043356786129}, {"Real Matrix Element"=-8.77825528387895, "Real Matrix Element"=6.120970543813109}, {"Real Matrix Element"=-8.72906856100395, "Real Matrix Element"=5.960061793131511}, {"Real Matrix Element"=-8.748557860702135, "Real Matrix Element"=5.620124078293323}, {"Real Matrix Element"=-8.565803169640153, "Real Matrix Element"=5.773663989947377}, {"Real Matrix Element"=-8.490520820406994, "Real Matrix Element"=5.700308490137754}, {"Real Matrix Element"=-8.563083394843693, "Real Matrix Element"=5.5283156067442825}, {"Real Matrix Element"=-8.716198427935314, "Real Matrix Element"=5.559196494624349}, {"Real Matrix Element"=-8.581444451256537, "Real Matrix Element"=5.653236331398812}, {"Real Matrix Element"=-8.36566398854045, "Real Matrix Element"=5.3834071989512005}, {"Real Matrix Element"=-8.304390119533547, "Real Matrix Element"=5.397609628104233}, {"Real Matrix Element"=-8.35995914551457, "Real Matrix Element"=5.086554756923889}, {"Real Matrix Element"=-8.300457583027601, "Real Matrix Element"=5.172978125580158}, {"Real Matrix Element"=-8.206472511177024, "Real Matrix Element"=5.020079577673998}, {"Real Matrix Element"=-8.17339369232863, "Real Matrix Element"=5.073694855149623}, {"Real Matrix Element"=-8.05272696035978, "Real Matrix Element"=4.961073478862043}, {"Real Matrix Element"=-8.00735713468638, "Real Matrix Element"=4.582322387990284}, {"Real Matrix Element"=-8.118634960621934, "Real Matrix Element"=4.795692309924664}, {"Real Matrix Element"=-8.043076368087206, "Real Matrix Element"=4.74489015613023}, {"Real Matrix Element"=-7.93737772811197, "Real Matrix Element"=4.720977397905222}, {"Real Matrix Element"=-7.9044830491542575, "Real Matrix Element"=4.4526655595380635}, {"Real Matrix Element"=-7.805573512516909, "Real Matrix Element"=4.409106604745945}, {"Real Matrix Element"=-7.679887705584279, "Real Matrix Element"=4.335214447483325}, {"Real Matrix Element"=-7.6688811835933475, "Real Matrix Element"=3.842270510470729}, {"Real Matrix Element"=-7.6558432102892695, "Real Matrix Element"=3.8921841645772717}, {"Real Matrix Element"=-7.498432930567476, "Real Matrix Element"=3.927951803302802}, {"Real Matrix Element"=-7.636077113239516, "Real Matrix Element"=3.771427939941814}, {"Real Matrix Element"=-7.543654343788005, "Real Matrix Element"=3.9442032991242724}, {"Real Matrix Element"=-7.440296941000858, "Real Matrix Element"=3.956536173171419}, {"Real Matrix Element"=-7.336565045884294, "Real Matrix Element"=4.040247829734623}, {"Real Matrix Element"=-7.388908634227123, "Real Matrix Element"=3.9189826480971464}, {"Real Matrix Element"=-7.3534553188639125, "Real Matrix Element"=3.6052741762232907}, {"Real Matrix Element"=-7.167478224119197, "Real Matrix Element"=3.5034963859845325}, {"Real Matrix Element"=-7.107612477291238, "Real Matrix Element"=3.4137340496400856}, {"Real Matrix Element"=-7.012696310668334, "Real Matrix Element"=3.3009121929152943}, {"Real Matrix Element"=-6.992535507661323, "Real Matrix Element"=3.2825490838916096}, {"Real Matrix Element"=-7.013541152213282, "Real Matrix Element"=3.2113057069253137}, {"Real Matrix Element"=-7.1908818430100485, "Real Matrix Element"=2.7411221442919786}, {"Real Matrix Element"=-7.142585020105198, "Real Matrix Element"=2.9367442405405875}, {"Real Matrix Element"=-7.1070191375453495, "Real Matrix Element"=2.8365982895989834}, {"Real Matrix Element"=-7.173255782826504, "Real Matrix Element"=2.7933658088552242}, {"Real Matrix Element"=-6.943204071424037, "Real Matrix Element"=2.995286344671341}, {"Real Matrix Element"=-6.732124941062728, "Real Matrix Element"=3.1832556212588408}, {"Real Matrix Element"=-6.616914535156143, "Real Matrix Element"=2.872685875058332}, {"Real Matrix Element"=-6.6446713166624, "Real Matrix Element"=2.6166909017349034}, {"Real Matrix Element"=-6.552149990612152, "Real Matrix Element"=2.6184942124723127}, {"Real Matrix Element"=-6.378507892361211, "Real Matrix Element"=2.9005872875441767}, {"Real Matrix Element"=-6.298676740555, "Real Matrix Element"=2.7463330050784243}, {"Real Matrix Element"=-6.308185271013789, "Real Matrix Element"=2.361617677275038}, {"Real Matrix Element"=-6.194981074515892, "Real Matrix Element"=2.390362201777021}, {"Real Matrix Element"=-6.246785602525975, "Real Matrix Element"=2.2149449807298693}, {"Real Matrix Element"=-6.164475975886344, "Real Matrix Element"=2.233383791351185}, {"Real Matrix Element"=-6.104017112431644, "Real Matrix Element"=2.164240024148063}, {"Real Matrix Element"=-6.104922884782478, "Real Matrix Element"=2.073242866667716}, {"Real Matrix Element"=-6.034395007553381, "Real Matrix Element"=2.0039663492839628}, {"Real Matrix Element"=-5.997660573592598, "Real Matrix Element"=1.756253973426315}, {"Real Matrix Element"=-5.985809061077896, "Real Matrix Element"=1.665004483087911}, {"Real Matrix Element"=-5.872676778922834, "Real Matrix Element"=1.804207357428839}, {"Real Matrix Element"=-5.764420859634181, "Real Matrix Element"=1.7759466741033851}, {"Real Matrix Element"=-5.642078661273526, "Real Matrix Element"=1.8227654830367417}, {"Real Matrix Element"=-5.649528546219241, "Real Matrix Element"=1.723824709075247}, {"Real Matrix Element"=-5.612366983285412, "Real Matrix Element"=1.499950768305231}, {"Real Matrix Element"=-5.527526583219875, "Real Matrix Element"=1.7379111943410253}, {"Real Matrix Element"=-5.541395701394104, "Real Matrix Element"=1.5705378440285387}, {"Real Matrix Element"=-5.441692185287382, "Real Matrix Element"=1.7026515175804142}, {"Real Matrix Element"=-5.333647013851528, "Real Matrix Element"=1.683723829502288}, {"Real Matrix Element"=-5.372303065358384, "Real Matrix Element"=1.221708091675515}, {"Real Matrix Element"=-5.335275268780659, "Real Matrix Element"=1.2559507226499962}, {"Real Matrix Element"=-5.1980797333357875, "Real Matrix Element"=1.1994330634200094}, {"Real Matrix Element"=-4.94718008503043, "Real Matrix Element"=1.5107488876040367}, {"Real Matrix Element"=-4.919088042289519, "Real Matrix Element"=1.5200756031923395}, {"Real Matrix Element"=-4.877930918521491, "Real Matrix Element"=1.1124056423612432}, {"Real Matrix Element"=-4.847727901600941, "Real Matrix Element"=1.2261172837321626}, {"Real Matrix Element"=-4.7689277555024825, "Real Matrix Element"=0.8139393491096261}, {"Real Matrix Element"=-4.65752181281426, "Real Matrix Element"=1.21187358670209}, {"Real Matrix Element"=-4.59003790656814, "Real Matrix Element"=0.9932341665652347}, {"Real Matrix Element"=-4.538212203821052, "Real Matrix Element"=0.6556265156399019}, {"Real Matrix Element"=-4.451334255038585, "Real Matrix Element"=0.7188112194223267}, {"Real Matrix Element"=-4.3628997243690835, "Real Matrix Element"=0.638995596537203}, {"Real Matrix Element"=-4.185241316692764, "Real Matrix Element"=0.954516703401068}, {"Real Matrix Element"=-4.155585082162706, "Real Matrix Element"=0.7015840964533057}, {"Real Matrix Element"=-4.051690237686029, "Real Matrix Element"=0.7533743865001095}, {"Real Matrix Element"=-3.9671383619289227, "Real Matrix Element"=0.6925998114703162}, {"Real Matrix Element"=-3.872798215011389, "Real Matrix Element"=0.7104255731443514}, {"Real Matrix Element"=-3.745895322658133, "Real Matrix Element"=0.7422051740725859}, {"Real Matrix Element"=-3.7146827217358562, "Real Matrix Element"=0.3869155512203065}, {"Real Matrix Element"=-3.6276476745064605, "Real Matrix Element"=0.6361649554060685}, {"Real Matrix Element"=-3.4849085682028527, "Real Matrix Element"=0.7171838229454518}, {"Real Matrix Element"=-3.3611289620349782, "Real Matrix Element"=0.9516376419737147}, {"Real Matrix Element"=-3.283723438801893, "Real Matrix Element"=1.0466287224618438}, {"Real Matrix Element"=-3.2241466553029325, "Real Matrix Element"=1.050063744188248}, {"Real Matrix Element"=-3.154866839449764, "Real Matrix Element"=1.1423527579694013}, {"Real Matrix Element"=-3.072653730370749, "Real Matrix Element"=1.033799127790837}, {"Real Matrix Element"=-3.0388585293294668, "Real Matrix Element"=0.9088836611298898}, {"Real Matrix Element"=-3.0316204327459273, "Real Matrix Element"=0.5511292282651759}, {"Real Matrix Element"=-2.9811525511114776, "Real Matrix Element"=0.6169863983845834}, {"Real Matrix Element"=-2.9025481991695847, "Real Matrix Element"=0.6878278479278678}, {"Real Matrix Element"=-2.804072166757793, "Real Matrix Element"=0.4372408921920774}, {"Real Matrix Element"=-2.7342974356427625, "Real Matrix Element"=0.31223787647654855}, {"Real Matrix Element"=-2.6675988677823956, "Real Matrix Element"=0.228647740468249}, {"Real Matrix Element"=-2.5808076732813734, "Real Matrix Element"=0.31532161756120536}, {"Real Matrix Element"=-2.518482880604688, "Real Matrix Element"=0.5233988871528935}, {"Real Matrix Element"=-2.4138059508306315, "Real Matrix Element"=0.2340259517179205}, {"Real Matrix Element"=-2.4147768280068256, "Real Matrix Element"=0.1043068589475597}, {"Real Matrix Element"=-2.2766016015976764, "Real Matrix Element"=0.05402720589995817}, {"Real Matrix Element"=-2.1393552279117802, "Real Matrix Element"=-0.004808778867342295}, {"Real Matrix Element"=-2.103710061693266, "Real Matrix Element"=0.30696235662434823}, {"Real Matrix Element"=-2.0511579903868746, "Real Matrix Element"=0.3965138944157577}, {"Real Matrix Element"=-2.025104463795925, "Real Matrix Element"=0.3742873206353112}, {"Real Matrix Element"=-1.9479222895900514, "Real Matrix Element"=0.32822309526040455}, {"Real Matrix Element"=-1.7997439355922777, "Real Matrix Element"=0.558946746083766}, {"Real Matrix Element"=-1.8409602378508332, "Real Matrix Element"=0.3303711472139087}, {"Real Matrix Element"=-1.7183884729311876, "Real Matrix Element"=0.32315665737414473}, {"Real Matrix Element"=-1.685978011265582, "Real Matrix Element"=0.14947406314274575}, {"Real Matrix Element"=-1.5880299395277246, "Real Matrix Element"=0.33917033879504077}, {"Real Matrix Element"=-1.5253010749016367, "Real Matrix Element"=0.3005058108838623}, {"Real Matrix Element"=-1.41156977806624, "Real Matrix Element"=0.45195188323135604}, {"Real Matrix Element"=-1.300047043479067, "Real Matrix Element"=0.2670188116311215}, {"Real Matrix Element"=-1.2702959539928216, "Real Matrix Element"=0.2352805426704716}, {"Real Matrix Element"=-1.1881842638641884, "Real Matrix Element"=0.38527590028312814}, {"Real Matrix Element"=-1.090547733571658, "Real Matrix Element"=0.1263892366740578}, {"Real Matrix Element"=-0.9499980445033663, "Real Matrix Element"=0.32893325729299916}, {"Real Matrix Element"=-0.7063358839830571, "Real Matrix Element"=0.5109177580636369}, {"Real Matrix Element"=-0.738700562969991, "Real Matrix Element"=0.6289941290451929}, {"Real Matrix Element"=-0.6882314105789197, "Real Matrix Element"=0.5193471689023086}, {"Real Matrix Element"=-0.5371046913980385, "Real Matrix Element"=0.5607181540575049}, {"Real Matrix Element"=-0.5148076161200097, "Real Matrix Element"=0.5309683181314114}, {"Real Matrix Element"=-0.3951191523295907, "Real Matrix Element"=0.6228328084901668}, {"Real Matrix Element"=-0.18456576064905755, "Real Matrix Element"=0.7300980360464411}, {"Real Matrix Element"=-0.2334372766504017, "Real Matrix Element"=0.8659158306756788}, {"Real Matrix Element"=-0.018309819125373883, "Real Matrix Element"=0.8885704334743475}, {"Real Matrix Element"=0.30377850528069306, "Real Matrix Element"=0.9829612396679788}, {"Real Matrix Element"=0.28780493250647543, "Real Matrix Element"=0.9249238315303528}, {"Real Matrix Element"=0.4589219051411653, "Real Matrix Element"=0.8805780676070799}, {"Real Matrix Element"=0.6414704216085696, "Real Matrix Element"=0.7816978654102004}, {"Real Matrix Element"=0.8416589252864348, "Real Matrix Element"=0.775135463249265}, {"Real Matrix Element"=1.1650041161975058, "Real Matrix Element"=0.7769195432783634}, {"Real Matrix Element"=1.5276064018404336, "Real Matrix Element"=0.6470691637773525}, {"Real Matrix Element"=1.6657312367760835, "Real Matrix Element"=0.4833059713440139}, {"Real Matrix Element"=1.8441120990031754, "Real Matrix Element"=0.34917505834867724}, {"Real Matrix Element"=2.021748326589091, "Real Matrix Element"=0.3054015901962532}, {"Real Matrix Element"=2.0147639338429553, "Real Matrix Element"=0.30859209194309184}, {"Real Matrix Element"=1.966591134013039, "Real Matrix Element"=0.28686828705172857}, {"Real Matrix Element"=2.043018003839024, "Real Matrix Element"=0.2233211474807893}, {"Real Matrix Element"=2.085956770936724, "Real Matrix Element"=0.21930038061424895}, {"Real Matrix Element"=2.2466770601941546, "Real Matrix Element"=0.11173899713349109}, {"Real Matrix Element"=2.3021407909998692, "Real Matrix Element"=0.10039010079664556}, {"Real Matrix Element"=2.1631548976525057, "Real Matrix Element"=0.18339466683633443}, {"Real Matrix Element"=2.2341292254464262, "Real Matrix Element"=0.09047644498316515}, {"Real Matrix Element"=2.427737623542115, "Real Matrix Element"=0.029624190963250675}, {"Real Matrix Element"=2.441111556111267, "Real Matrix Element"=0.044569022314116094}, {"Real Matrix Element"=2.5744846045952103, "Real Matrix Element"=-0.013773444218112843}, {"Real Matrix Element"=2.6244025390675816, "Real Matrix Element"=0.11653941140753349}, {"Real Matrix Element"=2.58551050067227, "Real Matrix Element"=0.04579140096199397}, {"Real Matrix Element"=2.659316457648961, "Real Matrix Element"=0.11716548979816321}, {"Real Matrix Element"=2.9230572954105756, "Real Matrix Element"=0.08857952026631674}, {"Real Matrix Element"=2.9737430556454556, "Real Matrix Element"=0.14415419610534036}, {"Real Matrix Element"=3.0088724046945785, "Real Matrix Element"=0.21962558760978512}, {"Real Matrix Element"=3.1479135992226097, "Real Matrix Element"=0.1269021949607978}, {"Real Matrix Element"=3.057741831168075, "Real Matrix Element"=0.24387817064370326}, {"Real Matrix Element"=3.3318518803487454, "Real Matrix Element"=0.16473110845874567}, {"Real Matrix Element"=3.3741512656168107, "Real Matrix Element"=0.16159241101023547}, {"Real Matrix Element"=3.5475390922052497, "Real Matrix Element"=0.1621649752958614}, {"Real Matrix Element"=3.585058760476445, "Real Matrix Element"=0.31231265492464577}, {"Real Matrix Element"=3.8031784955971504, "Real Matrix Element"=0.27828397604110344}, {"Real Matrix Element"=4.176278379338662, "Real Matrix Element"=0.27622487635031795}, {"Real Matrix Element"=4.320570652558516, "Real Matrix Element"=0.25055902934006463}, {"Real Matrix Element"=4.31012469980914, "Real Matrix Element"=0.2726976476050805}, {"Real Matrix Element"=4.227732318907376, "Real Matrix Element"=0.36968510816801897}, {"Real Matrix Element"=4.291237237780053, "Real Matrix Element"=0.5099333022642477}, {"Real Matrix Element"=4.359154048442046, "Real Matrix Element"=0.5655779379089643}, {"Real Matrix Element"=4.610955020585241, "Real Matrix Element"=0.6967329121198996}, {"Real Matrix Element"=4.721786802577094, "Real Matrix Element"=0.7670620033969657}, {"Real Matrix Element"=4.805319741266692, "Real Matrix Element"=0.8456370528910289}, {"Real Matrix Element"=4.907874758974723, "Real Matrix Element"=0.9672047790755748}, {"Real Matrix Element"=5.086963878592098, "Real Matrix Element"=1.0060083974200331}, {"Real Matrix Element"=5.207130346633222, "Real Matrix Element"=1.0615960823449406}, {"Real Matrix Element"=5.157344205020074, "Real Matrix Element"=1.1523324485464703}, {"Real Matrix Element"=5.335647853216283, "Real Matrix Element"=1.1729084134271586}, {"Real Matrix Element"=5.405081461950799, "Real Matrix Element"=1.2775403261522031}, {"Real Matrix Element"=5.488597648988109, "Real Matrix Element"=1.3463068035872747}, {"Real Matrix Element"=5.541232779386242, "Real Matrix Element"=1.3933747708393651}, {"Real Matrix Element"=5.661036238137651, "Real Matrix Element"=1.464743465575102}, {"Real Matrix Element"=5.8561870121331845, "Real Matrix Element"=1.5095606089980438}, {"Real Matrix Element"=5.900712935820929, "Real Matrix Element"=1.6041085072817696}, {"Real Matrix Element"=5.92909387672455, "Real Matrix Element"=1.6943062687444101}, {"Real Matrix Element"=6.249629525187588, "Real Matrix Element"=1.7839238387113234}, {"Real Matrix Element"=6.216698131916994, "Real Matrix Element"=1.8507075391067125}, {"Real Matrix Element"=6.1602793068987705, "Real Matrix Element"=1.8276436808987206}, {"Real Matrix Element"=6.157247352686177, "Real Matrix Element"=1.9768877506109606}, {"Real Matrix Element"=6.335994033969795, "Real Matrix Element"=2.1541991097023847}, {"Real Matrix Element"=6.385312655741874, "Real Matrix Element"=2.266602052490795}, {"Real Matrix Element"=6.462137762720645, "Real Matrix Element"=2.525357489850152}, {"Real Matrix Element"=6.560385576631828, "Real Matrix Element"=2.6444054492924964}, {"Real Matrix Element"=6.6912604877494815, "Real Matrix Element"=2.853456490662136}, {"Real Matrix Element"=6.728647994205898, "Real Matrix Element"=2.9655481373688644}, {"Real Matrix Element"=6.844819050333562, "Real Matrix Element"=3.0327145981914727}, {"Real Matrix Element"=6.965475055762987, "Real Matrix Element"=3.20696905152826}, {"Real Matrix Element"=7.007174614462419, "Real Matrix Element"=3.2160194257728074}, {"Real Matrix Element"=7.128521793585396, "Real Matrix Element"=3.3012746564706617}, {"Real Matrix Element"=7.175391229803522, "Real Matrix Element"=3.383265737101154}, {"Real Matrix Element"=7.186979122464782, "Real Matrix Element"=3.3815763117031006}, {"Real Matrix Element"=7.306672074548062, "Real Matrix Element"=3.574136271233444}, {"Real Matrix Element"=7.332564926550973, "Real Matrix Element"=3.6062120649247027}, {"Real Matrix Element"=7.219076696219226, "Real Matrix Element"=3.6555353977428524}, {"Real Matrix Element"=7.250477749663124, "Real Matrix Element"=3.6972059491746774}, {"Real Matrix Element"=7.338683491413695, "Real Matrix Element"=3.7082274495306313}, {"Real Matrix Element"=7.353749570607225, "Real Matrix Element"=3.6986001930237866}, {"Real Matrix Element"=7.612526692941833, "Real Matrix Element"=3.5985449959032167}, {"Real Matrix Element"=7.651672933945467, "Real Matrix Element"=3.614690616501432}, {"Real Matrix Element"=7.728496926345336, "Real Matrix Element"=3.5778944338705845}, {"Real Matrix Element"=7.561440429449951, "Real Matrix Element"=3.6376127066828547}, {"Real Matrix Element"=7.675998485917753, "Real Matrix Element"=3.724244529356748}, {"Real Matrix Element"=7.644861502228955, "Real Matrix Element"=3.7399537009195254}, {"Real Matrix Element"=7.480418394838927, "Real Matrix Element"=3.915517291087263}, {"Real Matrix Element"=7.434997920433176, "Real Matrix Element"=3.875447102797714}, {"Real Matrix Element"=7.633575343181837, "Real Matrix Element"=3.81142654767513}, {"Real Matrix Element"=7.449539433464316, "Real Matrix Element"=3.903779151256584}, {"Real Matrix Element"=7.434300876835795, "Real Matrix Element"=4.008330316980462}, {"Real Matrix Element"=7.559642777873894, "Real Matrix Element"=4.005103396803676}, {"Real Matrix Element"=7.578804499078848, "Real Matrix Element"=4.070593709905861}, {"Real Matrix Element"=7.804774824183092, "Real Matrix Element"=4.045334056596868}, {"Real Matrix Element"=8.061894338639144, "Real Matrix Element"=4.058502921997579}, {"Real Matrix Element"=8.071632901800289, "Real Matrix Element"=4.131741724066153}, {"Real Matrix Element"=8.287432967345785, "Real Matrix Element"=4.197404374255615}, {"Real Matrix Element"=8.09326476835726, "Real Matrix Element"=4.293724807038494}, {"Real Matrix Element"=8.067799025093244, "Real Matrix Element"=4.4345980872126}, {"Real Matrix Element"=8.119042552066606, "Real Matrix Element"=4.534604579754017}, {"Real Matrix Element"=8.077876640375978, "Real Matrix Element"=4.638706703473464}, {"Real Matrix Element"=8.158391173709875, "Real Matrix Element"=4.668267502124541}, {"Real Matrix Element"=8.18341150495798, "Real Matrix Element"=4.750160893852613}, {"Real Matrix Element"=8.247620165054785, "Real Matrix Element"=4.764147286551949}, {"Real Matrix Element"=8.281632569772016, "Real Matrix Element"=4.912371330206761}, {"Real Matrix Element"=8.464610578676316, "Real Matrix Element"=4.924454548987411}, {"Real Matrix Element"=8.402361188206926, "Real Matrix Element"=5.105674716653764}, {"Real Matrix Element"=8.791310532657736, "Real Matrix Element"=5.370423860316536}, {"Real Matrix Element"=9.027479020134653, "Real Matrix Element"=5.553864651821163}, {"Real Matrix Element"=9.137157242934117, "Real Matrix Element"=5.858493350373172}, {"Real Matrix Element"=9.18562065540263, "Real Matrix Element"=5.968436837409526}, {"Real Matrix Element"=9.13454052829577, "Real Matrix Element"=6.127486449524582}, {"Real Matrix Element"=9.451096304689377, "Real Matrix Element"=6.380899226896659}, {"Real Matrix Element"=9.395459589646897, "Real Matrix Element"=6.478025158837784}, {"Real Matrix Element"=9.435540321339296, "Real Matrix Element"=6.601011844666219}, {"Real Matrix Element"=9.614671444373016, "Real Matrix Element"=6.6967792681583145}, {"Real Matrix Element"=9.461114738940847, "Real Matrix Element"=6.6961617137648135}, {"Real Matrix Element"=9.323909456801038, "Real Matrix Element"=6.729066956793637}, {"Real Matrix Element"=9.473397496048646, "Real Matrix Element"=6.746740047769825}, {"Real Matrix Element"=9.399212575541032, "Real Matrix Element"=6.824665080802258}, {"Real Matrix Element"=9.345238169731909, "Real Matrix Element"=6.809581814300138}, {"Real Matrix Element"=9.131478182629547, "Real Matrix Element"=7.052673895275924}, {"Real Matrix Element"=9.311895623709, "Real Matrix Element"=6.965632574076661}, {"Real Matrix Element"=9.317039738358089, "Real Matrix Element"=7.106004688672617}, {"Real Matrix Element"=9.325364553097195, "Real Matrix Element"=7.161189456949826}, {"Real Matrix Element"=9.288951653761838, "Real Matrix Element"=7.2305985559714605}, {"Real Matrix Element"=9.360404509365265, "Real Matrix Element"=7.265053598015139}, {"Real Matrix Element"=9.288360514358313, "Real Matrix Element"=7.370016359351302}, {"Real Matrix Element"=9.200658570994854, "Real Matrix Element"=7.485995987146842}, {"Real Matrix Element"=9.33339843765502, "Real Matrix Element"=7.494998862477568}, {"Real Matrix Element"=9.539379926300454, "Real Matrix Element"=7.4626451309071555}, {"Real Matrix Element"=9.565059796096735, "Real Matrix Element"=7.565243890347254}, {"Real Matrix Element"=9.681364684686585, "Real Matrix Element"=7.713821510421394}, {"Real Matrix Element"=9.653377380926406, "Real Matrix Element"=7.76156990210144}, {"Real Matrix Element"=9.6218701278617, "Real Matrix Element"=7.875181086568654}, {"Real Matrix Element"=9.441956198623751, "Real Matrix Element"=7.974672835114378}, {"Real Matrix Element"=9.654932506631772, "Real Matrix Element"=8.073384691174175}, {"Real Matrix Element"=9.755615230755897, "Real Matrix Element"=8.213542124507951}, {"Real Matrix Element"=9.744295194471317, "Real Matrix Element"=8.313285940784601}, {"Real Matrix Element"=9.620990024080628, "Real Matrix Element"=8.360156906773943}, {"Real Matrix Element"=9.72329700765277, "Real Matrix Element"=8.483948312977182}, {"Real Matrix Element"=9.706190631137977, "Real Matrix Element"=8.614553365353594}, {"Real Matrix Element"=9.696637358447786, "Real Matrix Element"=8.748453496109413}, {"Real Matrix Element"=9.838519887025631, "Real Matrix Element"=8.8061422233634}, {"Real Matrix Element"=9.81079638493081, "Real Matrix Element"=8.897053386357436}, {"Real Matrix Element"=9.895362336219543, "Real Matrix Element"=9.002981652565012}, {"Real Matrix Element"=9.81505380580012, "Real Matrix Element"=9.117643117376035}, {"Real Matrix Element"=9.97523641078563, "Real Matrix Element"=9.29062561634402}, {"Real Matrix Element"=10.236553141967281, "Real Matrix Element"=9.515426219326192}, {"Real Matrix Element"=10.143054797804096, "Real Matrix Element"=9.659326736368007}, {"Real Matrix Element"=10.195353868252658, "Real Matrix Element"=9.853818439791734}, {"Real Matrix Element"=10.131130939988502, "Real Matrix Element"=10.194947994586954}, {"Real Matrix Element"=10.20577125598272, "Real Matrix Element"=10.337103932775038}, {"Real Matrix Element"=10.293015967965566, "Real Matrix Element"=10.36155219160318}, {"Real Matrix Element"=10.370324097429851, "Real Matrix Element"=10.506325254727162}, {"Real Matrix Element"=10.287444192368591, "Real Matrix Element"=10.584374657937586}, {"Real Matrix Element"=9.99178812816685, "Real Matrix Element"=10.514500722294063}, {"Real Matrix Element"=9.866119760446834, "Real Matrix Element"=10.545697931809574}, {"Real Matrix Element"=9.872193335517647, "Real Matrix Element"=10.603831580781657}, {"Real Matrix Element"=9.754343185919865, "Real Matrix Element"=10.70039645855139}, {"Real Matrix Element"=9.839274256294443, "Real Matrix Element"=10.830929702696661}, {"Real Matrix Element"=9.603408156236581, "Real Matrix Element"=10.88996318665285}, {"Real Matrix Element"=9.812434701521529, "Real Matrix Element"=11.019451111764178}, {"Real Matrix Element"=9.935708221986749, "Real Matrix Element"=11.085824989804694}, {"Real Matrix Element"=9.690136929360712, "Real Matrix Element"=11.265153167379216}, {"Real Matrix Element"=9.63354004847201, "Real Matrix Element"=11.280304559626723}, {"Real Matrix Element"=9.5738178592244, "Real Matrix Element"=11.264233951428901}, {"Real Matrix Element"=9.46061666883795, "Real Matrix Element"=11.34699761818162}, {"Real Matrix Element"=9.300015560527179, "Real Matrix Element"=11.502685954071861}, {"Real Matrix Element"=9.32691153111023, "Real Matrix Element"=11.533039146447239}, {"Real Matrix Element"=9.279012885321741, "Real Matrix Element"=11.539769672511724}, {"Real Matrix Element"=9.078922750748879, "Real Matrix Element"=11.689286491016455}, {"Real Matrix Element"=9.285400157190002, "Real Matrix Element"=11.767418328280291}, {"Real Matrix Element"=9.339735595277164, "Real Matrix Element"=11.793378579131254}, {"Real Matrix Element"=9.201064014736792, "Real Matrix Element"=11.949772011612593}, {"Real Matrix Element"=9.48455877786939, "Real Matrix Element"=12.012787625956944}, {"Real Matrix Element"=9.670614005660719, "Real Matrix Element"=12.173586032386485}, {"Real Matrix Element"=9.70419119367051, "Real Matrix Element"=12.441416652778683}, {"Real Matrix Element"=9.472579313654832, "Real Matrix Element"=12.566885027340353}, {"Real Matrix Element"=9.694546528620046, "Real Matrix Element"=12.7140695185492}, {"Real Matrix Element"=9.631426587128937, "Real Matrix Element"=12.906307142476216}, {"Real Matrix Element"=9.6316620797809, "Real Matrix Element"=13.000537646701554}, {"Real Matrix Element"=9.381508402599517, "Real Matrix Element"=13.085451366633267}, {"Real Matrix Element"=9.091609494881265, "Real Matrix Element"=13.195872284441247}, {"Real Matrix Element"=9.191259955265272, "Real Matrix Element"=13.378902222249254}, {"Real Matrix Element"=9.285920545707107, "Real Matrix Element"=13.478541500570229}, {"Real Matrix Element"=9.206811809766757, "Real Matrix Element"=13.496631542527254}, {"Real Matrix Element"=9.122703971855284, "Real Matrix Element"=13.531155858287345}, {"Real Matrix Element"=9.184913281419684, "Real Matrix Element"=13.740111546045783}, {"Real Matrix Element"=8.865162858778055, "Real Matrix Element"=13.818774636480859}, {"Real Matrix Element"=8.853846775633668, "Real Matrix Element"=13.940069032633547}, {"Real Matrix Element"=8.853222982269962, "Real Matrix Element"=14.075732027145046}, {"Real Matrix Element"=8.966804194536657, "Real Matrix Element"=14.135648034479297}, {"Real Matrix Element"=9.085226035301746, "Real Matrix Element"=14.161084268491782}, {"Real Matrix Element"=8.849416756011204, "Real Matrix Element"=14.234842713929366}, {"Real Matrix Element"=9.03631712448827, "Real Matrix Element"=14.305856445386738}, {"Real Matrix Element"=8.937030710838595, "Real Matrix Element"=14.359175896574937}, {"Real Matrix Element"=8.715344023496112, "Real Matrix Element"=14.484084260144233}, {"Real Matrix Element"=8.576830453167943, "Real Matrix Element"=14.527702039601191}, {"Real Matrix Element"=8.499537989744077, "Real Matrix Element"=14.458537337902827}, {"Real Matrix Element"=8.367621737354726, "Real Matrix Element"=14.66381051398132}, {"Real Matrix Element"=8.157001658854913, "Real Matrix Element"=14.802950290358599}, {"Real Matrix Element"=8.290473645248914, "Real Matrix Element"=14.751253149137927}, {"Real Matrix Element"=8.09427500599427, "Real Matrix Element"=14.862340227706593}, {"Real Matrix Element"=7.999099406037615, "Real Matrix Element"=15.042383414490892}, {"Real Matrix Element"=8.033196177641164, "Real Matrix Element"=15.028300428586043}, {"Real Matrix Element"=7.822095139911754, "Real Matrix Element"=15.147938552245435}, {"Real Matrix Element"=7.800508923817574, "Real Matrix Element"=15.203597097750094}, {"Real Matrix Element"=7.768209114004175, "Real Matrix Element"=15.276475103805172}, {"Real Matrix Element"=7.91184685325973, "Real Matrix Element"=15.348685319787576}, {"Real Matrix Element"=7.92609360062375, "Real Matrix Element"=15.44247027820673}, {"Real Matrix Element"=7.6791672905541155, "Real Matrix Element"=15.496490037639761}, {"Real Matrix Element"=7.658568836113813, "Real Matrix Element"=15.589517840356754}, {"Real Matrix Element"=7.672359754056809, "Real Matrix Element"=15.68239118425632}, {"Real Matrix Element"=7.702643597310469, "Real Matrix Element"=15.760208159836655}, {"Real Matrix Element"=7.7516071422285915, "Real Matrix Element"=15.832250448744546}, {"Real Matrix Element"=7.66697229886697, "Real Matrix Element"=15.895942255326869}, {"Real Matrix Element"=7.763421395828019, "Real Matrix Element"=15.927457040474406}, {"Real Matrix Element"=7.539771114349705, "Real Matrix Element"=16.035069751538966}, {"Real Matrix Element"=7.4716148470198025, "Real Matrix Element"=16.141259538570996}, {"Real Matrix Element"=7.4159006560251415, "Real Matrix Element"=16.25713572374613}, {"Real Matrix Element"=7.277268786393869, "Real Matrix Element"=16.441303437441032}, {"Real Matrix Element"=7.227228456275255, "Real Matrix Element"=16.491969265973243}, {"Real Matrix Element"=7.338998527318836, "Real Matrix Element"=16.468589884289745}, {"Real Matrix Element"=7.340511290429183, "Real Matrix Element"=16.467925677919304}, {"Real Matrix Element"=7.105275159688695, "Real Matrix Element"=16.560035561060886}, {"Real Matrix Element"=6.991726667685064, "Real Matrix Element"=16.568561872180695}, {"Real Matrix Element"=6.879482705040036, "Real Matrix Element"=16.64278200943879}, {"Real Matrix Element"=6.694987168993432, "Real Matrix Element"=16.798680554582944}, {"Real Matrix Element"=6.519361404612029, "Real Matrix Element"=17.009443815944138}, {"Real Matrix Element"=6.312010871397966, "Real Matrix Element"=17.158899758514224}, {"Real Matrix Element"=6.215467585456371, "Real Matrix Element"=17.383151261162812}, {"Real Matrix Element"=6.119861922501692, "Real Matrix Element"=17.524208503524058}, {"Real Matrix Element"=6.062020165971798, "Real Matrix Element"=17.376852061815868}, {"Real Matrix Element"=6.230903633303492, "Real Matrix Element"=17.25628571413896}, {"Real Matrix Element"=6.037331501960522, "Real Matrix Element"=17.2305722215827}, {"Real Matrix Element"=6.099871134559044, "Real Matrix Element"=17.335634715091043}, {"Real Matrix Element"=6.117396283925198, "Real Matrix Element"=17.36246096411416}, {"Real Matrix Element"=5.891808363082865, "Real Matrix Element"=17.659990081063427}, {"Real Matrix Element"=5.803274159028717, "Real Matrix Element"=17.746863836977806}, {"Real Matrix Element"=5.709675333290001, "Real Matrix Element"=17.70488206699843}, {"Real Matrix Element"=5.632780171637595, "Real Matrix Element"=17.874763249818304}, {"Real Matrix Element"=5.454256673104699, "Real Matrix Element"=17.958074721771517}, {"Real Matrix Element"=5.445198007935964, "Real Matrix Element"=17.93168040874259}, {"Real Matrix Element"=5.495658092879441, "Real Matrix Element"=18.013455480412002}, {"Real Matrix Element"=5.424644870979695, "Real Matrix Element"=18.085053734122592}, {"Real Matrix Element"=5.238716295214582, "Real Matrix Element"=18.30674347261133}, {"Real Matrix Element"=5.123360170187024, "Real Matrix Element"=18.47660597594952}, {"Real Matrix Element"=5.159689591264228, "Real Matrix Element"=18.218183510039253}, {"Real Matrix Element"=5.118159469791317, "Real Matrix Element"=18.200759794341558}, {"Real Matrix Element"=5.064889433854732, "Real Matrix Element"=18.502564988953264}, {"Real Matrix Element"=5.064911446450237, "Real Matrix Element"=18.62276247585897}, {"Real Matrix Element"=4.727796903688105, "Real Matrix Element"=18.858289110727565}, {"Real Matrix Element"=4.781657446919913, "Real Matrix Element"=18.543870882292094}, {"Real Matrix Element"=4.807556425391776, "Real Matrix Element"=18.364886626186603}, {"Real Matrix Element"=4.620837275683193, "Real Matrix Element"=18.80775296007847}, {"Real Matrix Element"=4.498198786803636, "Real Matrix Element"=18.784314435378064}, {"Real Matrix Element"=4.365079169599265, "Real Matrix Element"=18.729173504492945}, {"Real Matrix Element"=4.160932466849765, "Real Matrix Element"=18.693726359435065}, {"Real Matrix Element"=4.002210738708911, "Real Matrix Element"=18.763126463361242}, {"Real Matrix Element"=4.015037828215928, "Real Matrix Element"=18.720880037498965}, {"Real Matrix Element"=3.894736536869436, "Real Matrix Element"=18.766556576437125}, {"Real Matrix Element"=3.920830553676393, "Real Matrix Element"=18.555371861506607}, {"Real Matrix Element"=3.7468948366199943, "Real Matrix Element"=18.821121379636672}, {"Real Matrix Element"=3.576245617978572, "Real Matrix Element"=18.904532531218635}, {"Real Matrix Element"=3.6708571185515755, "Real Matrix Element"=18.98552080717036}, {"Real Matrix Element"=3.631489114159884, "Real Matrix Element"=19.099692088894987}, {"Real Matrix Element"=3.6210680510665196, "Real Matrix Element"=19.215689256277983}, {"Real Matrix Element"=3.4839820865016184, "Real Matrix Element"=19.40363289352215}, {"Real Matrix Element"=3.481728406753725, "Real Matrix Element"=19.484201896313383}, {"Real Matrix Element"=3.4252023226221984, "Real Matrix Element"=19.651553683383103}, {"Real Matrix Element"=3.436354781896603, "Real Matrix Element"=19.409707755241982}, {"Real Matrix Element"=3.3405336640984755, "Real Matrix Element"=19.47591868855012}, {"Real Matrix Element"=3.2851667173061427, "Real Matrix Element"=19.317399013763662}, {"Real Matrix Element"=3.144148914244289, "Real Matrix Element"=19.68036818336485}, {"Real Matrix Element"=2.9832483610906935, "Real Matrix Element"=19.601804282470244}, {"Real Matrix Element"=2.9037266637601618, "Real Matrix Element"=19.519851649345476}, {"Real Matrix Element"=2.68766939797238, "Real Matrix Element"=19.334683461032874}, {"Real Matrix Element"=2.7476373180932727, "Real Matrix Element"=19.374806933605583}, {"Real Matrix Element"=2.4985346732449996, "Real Matrix Element"=19.453194852933436}, {"Real Matrix Element"=2.4183343539463436, "Real Matrix Element"=19.806357953410092}, {"Real Matrix Element"=2.4718294806116736, "Real Matrix Element"=19.72909566307848}, {"Real Matrix Element"=2.246129156197959, "Real Matrix Element"=19.95470351261662}, {"Real Matrix Element"=2.2233340697593986, "Real Matrix Element"=19.929584240174854}, {"Real Matrix Element"=2.19914958639723, "Real Matrix Element"=19.834332017345012}, {"Real Matrix Element"=2.111593624216784, "Real Matrix Element"=19.830064666445086}, {"Real Matrix Element"=1.9431310191230744, "Real Matrix Element"=19.764697837295834}, {"Real Matrix Element"=1.776532755076367, "Real Matrix Element"=19.66760137258149}, {"Real Matrix Element"=1.6609874227785935, "Real Matrix Element"=19.696792197184934}, {"Real Matrix Element"=1.4932439803658457, "Real Matrix Element"=19.731464170197775}, {"Real Matrix Element"=1.4728888528169786, "Real Matrix Element"=19.778267851583525}, {"Real Matrix Element"=1.4607861759909504, "Real Matrix Element"=19.698653187854475}, {"Real Matrix Element"=1.4026588838705893, "Real Matrix Element"=20.02578391706026}, {"Real Matrix Element"=1.2776581183745244, "Real Matrix Element"=19.898848292287678}, {"Real Matrix Element"=1.2243440177730425, "Real Matrix Element"=19.690191758186323}, {"Real Matrix Element"=1.159622376804089, "Real Matrix Element"=19.73673710537598}, {"Real Matrix Element"=1.0476878514261088, "Real Matrix Element"=19.306182574658475}, {"Real Matrix Element"=0.9929569313980762, "Real Matrix Element"=19.9397176346009}, {"Real Matrix Element"=0.8571030419226731, "Real Matrix Element"=20.015029797576855}, {"Real Matrix Element"=0.8037571205266882, "Real Matrix Element"=19.855130684894338}, {"Real Matrix Element"=0.7302053050167598, "Real Matrix Element"=19.743545913168635}, {"Real Matrix Element"=0.6342388484241694, "Real Matrix Element"=19.735572926682018}, {"Real Matrix Element"=0.5388674777970085, "Real Matrix Element"=19.6408973069242}, {"Real Matrix Element"=0.49573813298991715, "Real Matrix Element"=19.73532721897991}, {"Real Matrix Element"=0.41703108506564596, "Real Matrix Element"=20.002561775069392}, {"Real Matrix Element"=0.36136660372003937, "Real Matrix Element"=20.116245746213732}, {"Real Matrix Element"=0.36067846583515767, "Real Matrix Element"=19.956215989639826}, {"Real Matrix Element"=0.26260681138073805, "Real Matrix Element"=20.048552405484195}, {"Real Matrix Element"=0.11969261017022315, "Real Matrix Element"=19.92305236296284}, {"Real Matrix Element"=0.041434692401191124, "Real Matrix Element"=19.690615723481873}, {"Real Matrix Element"=-0.10971183853886118, "Real Matrix Element"=19.832036743748464}, {"Real Matrix Element"=-0.20999468390688458, "Real Matrix Element"=19.780860829099307}, {"Real Matrix Element"=-0.27128326798771785, "Real Matrix Element"=19.55601290729223}, {"Real Matrix Element"=-0.37663985242275877, "Real Matrix Element"=19.838303098547176}, {"Real Matrix Element"=-0.53343999934841, "Real Matrix Element"=19.750284013513703}, {"Real Matrix Element"=-0.6388852399830633, "Real Matrix Element"=20.07514939962937}, {"Real Matrix Element"=-0.6532923372408727, "Real Matrix Element"=20.10284151612794}, {"Real Matrix Element"=-0.6975700066088946, "Real Matrix Element"=20.198811052288}, {"Real Matrix Element"=-0.7610843778165113, "Real Matrix Element"=20.169102534811522}, {"Real Matrix Element"=-0.8517409430249506, "Real Matrix Element"=19.968431200075983}, {"Real Matrix Element"=-1.00050093285658, "Real Matrix Element"=19.829217047523116}, {"Real Matrix Element"=-1.0891166295084274, "Real Matrix Element"=19.923840076594487}, {"Real Matrix Element"=-1.1753677215997287, "Real Matrix Element"=19.785107173517307}, {"Real Matrix Element"=-1.3061186276279824, "Real Matrix Element"=19.61389946430275}, {"Real Matrix Element"=-1.338152018401189, "Real Matrix Element"=19.719104898561095}, {"Real Matrix Element"=-1.475033381205643, "Real Matrix Element"=19.96029960052449}, {"Real Matrix Element"=-1.6000992251755843, "Real Matrix Element"=19.48331905860049}, {"Real Matrix Element"=-1.7368526405079057, "Real Matrix Element"=19.462220913503096}, {"Real Matrix Element"=-1.9199525480767106, "Real Matrix Element"=19.627038630195674}, {"Real Matrix Element"=-1.975051911862143, "Real Matrix Element"=19.348424473103705}, {"Real Matrix Element"=-2.0734638636716154, "Real Matrix Element"=19.553080011472463}, {"Real Matrix Element"=-2.2417176166357784, "Real Matrix Element"=19.592986293127108}, {"Real Matrix Element"=-2.2994341697808536, "Real Matrix Element"=19.36825598310044}, {"Real Matrix Element"=-2.365540026511837, "Real Matrix Element"=19.37276169791596}, {"Real Matrix Element"=-2.45386034473866, "Real Matrix Element"=19.36792140812751}, {"Real Matrix Element"=-2.535710889732652, "Real Matrix Element"=19.36511410933778}, {"Real Matrix Element"=-2.6581786356623973, "Real Matrix Element"=19.067929861675715}, {"Real Matrix Element"=-2.7040705006274215, "Real Matrix Element"=19.179282147401953}, {"Real Matrix Element"=-2.7651484963536714, "Real Matrix Element"=19.362556039922307}, {"Real Matrix Element"=-2.8257829863056556, "Real Matrix Element"=19.40178472531832}, {"Real Matrix Element"=-2.955261748941807, "Real Matrix Element"=19.267339706268547}, {"Real Matrix Element"=-2.9872055140776888, "Real Matrix Element"=19.139984194472877}, {"Real Matrix Element"=-3.0932086506532954, "Real Matrix Element"=19.065075604833705}, {"Real Matrix Element"=-3.152052053812852, "Real Matrix Element"=18.940021782501592}, {"Real Matrix Element"=-3.2174138580375615, "Real Matrix Element"=18.794096247952986}, {"Real Matrix Element"=-3.3254152215281483, "Real Matrix Element"=18.941650693493866}, {"Real Matrix Element"=-3.4545568587062534, "Real Matrix Element"=18.8709001464941}, {"Real Matrix Element"=-3.545938039631078, "Real Matrix Element"=18.896677693658262}, {"Real Matrix Element"=-3.611816226377125, "Real Matrix Element"=18.800294320474492}, {"Real Matrix Element"=-3.6797440336474136, "Real Matrix Element"=18.6692304188549}, {"Real Matrix Element"=-3.8134139312606194, "Real Matrix Element"=18.754461199455744}, {"Real Matrix Element"=-3.9164393894937546, "Real Matrix Element"=18.812535304123053}, {"Real Matrix Element"=-4.029546652661513, "Real Matrix Element"=18.840550540910016}, {"Real Matrix Element"=-4.144873482383738, "Real Matrix Element"=18.980232492682564}, {"Real Matrix Element"=-4.205897114204169, "Real Matrix Element"=19.030911477169635}, {"Real Matrix Element"=-4.25118912611665, "Real Matrix Element"=18.69207297433856}, {"Real Matrix Element"=-4.345440841258114, "Real Matrix Element"=18.619890494129052}, {"Real Matrix Element"=-4.334705738238112, "Real Matrix Element"=18.426976226297164}, {"Real Matrix Element"=-4.378558421941204, "Real Matrix Element"=18.649581652081075}, {"Real Matrix Element"=-4.396658774935922, "Real Matrix Element"=18.302844552707455}, {"Real Matrix Element"=-4.449771929907119, "Real Matrix Element"=18.419255714996524}, {"Real Matrix Element"=-4.523525590812433, "Real Matrix Element"=18.462805639445957}, {"Real Matrix Element"=-4.660870286479777, "Real Matrix Element"=18.54839363195886}, {"Real Matrix Element"=-4.6742275990039435, "Real Matrix Element"=18.486101309620235}, {"Real Matrix Element"=-4.712558013967, "Real Matrix Element"=18.35517139224557}, {"Real Matrix Element"=-4.794335882740191, "Real Matrix Element"=18.139923221309992}, {"Real Matrix Element"=-4.960704415391274, "Real Matrix Element"=18.474305926684664}, {"Real Matrix Element"=-4.965575557552839, "Real Matrix Element"=18.212316280605865}, {"Real Matrix Element"=-5.072155995486342, "Real Matrix Element"=18.44156039620907}, {"Real Matrix Element"=-5.159509662249989, "Real Matrix Element"=18.398353480036764}, {"Real Matrix Element"=-5.284262281423633, "Real Matrix Element"=18.34808653905916}, {"Real Matrix Element"=-5.308264776349867, "Real Matrix Element"=18.071967525103506}, {"Real Matrix Element"=-5.448445023102603, "Real Matrix Element"=18.29740709507758}, {"Real Matrix Element"=-5.397962847356634, "Real Matrix Element"=17.838400112891705}, {"Real Matrix Element"=-5.530239055943502, "Real Matrix Element"=17.77378240314273}, {"Real Matrix Element"=-5.583993218573467, "Real Matrix Element"=17.38775585885903}, {"Real Matrix Element"=-5.621349190671377, "Real Matrix Element"=17.423519450710735}, {"Real Matrix Element"=-5.646885543938781, "Real Matrix Element"=17.322790222975684}, {"Real Matrix Element"=-5.711917801703574, "Real Matrix Element"=17.319110324290687}, {"Real Matrix Element"=-5.753596589485114, "Real Matrix Element"=17.472488537186376}, {"Real Matrix Element"=-5.793583929047714, "Real Matrix Element"=17.43009445014323}, {"Real Matrix Element"=-5.872823096078534, "Real Matrix Element"=17.657220267944066}, {"Real Matrix Element"=-5.856695945315325, "Real Matrix Element"=17.047678718881386}, {"Real Matrix Element"=-5.988564552348745, "Real Matrix Element"=16.839969147826032}, {"Real Matrix Element"=-6.1186643992734595, "Real Matrix Element"=17.16317059646164}, {"Real Matrix Element"=-6.0789060836086195, "Real Matrix Element"=17.01699591832778}, {"Real Matrix Element"=-6.23771406793616, "Real Matrix Element"=17.11222863067157}, {"Real Matrix Element"=-6.23340496623347, "Real Matrix Element"=17.04230957283262}, {"Real Matrix Element"=-6.198273099095893, "Real Matrix Element"=16.961806713010503}, {"Real Matrix Element"=-6.191600947943344, "Real Matrix Element"=16.569800733373693}, {"Real Matrix Element"=-6.3350755174485665, "Real Matrix Element"=16.84110384383744}, {"Real Matrix Element"=-6.271887195090419, "Real Matrix Element"=16.652104343343357}, {"Real Matrix Element"=-6.1709263100527245, "Real Matrix Element"=16.19702622973577}, {"Real Matrix Element"=-6.370471121480378, "Real Matrix Element"=16.550148981317122}, {"Real Matrix Element"=-6.416562422055308, "Real Matrix Element"=16.572504753812808}, {"Real Matrix Element"=-6.349424803560839, "Real Matrix Element"=16.39255359522436}, {"Real Matrix Element"=-6.400880676845481, "Real Matrix Element"=16.508841517641653}, {"Real Matrix Element"=-6.45805526049779, "Real Matrix Element"=16.440417489585393}, {"Real Matrix Element"=-6.597811946030432, "Real Matrix Element"=16.32411659610854}, {"Real Matrix Element"=-6.600599833781102, "Real Matrix Element"=16.12208063363312}, {"Real Matrix Element"=-6.574150276142064, "Real Matrix Element"=16.315002185047273}, {"Real Matrix Element"=-6.684895954350603, "Real Matrix Element"=16.242012832097426}, {"Real Matrix Element"=-6.82135400161416, "Real Matrix Element"=16.149307169274678}, {"Real Matrix Element"=-6.935296948633525, "Real Matrix Element"=15.865424251301864}, {"Real Matrix Element"=-6.850539522831134, "Real Matrix Element"=15.712601218858271}, {"Real Matrix Element"=-6.988678192060678, "Real Matrix Element"=15.724803080040989}, {"Real Matrix Element"=-7.060252151611846, "Real Matrix Element"=15.913546908226069}, {"Real Matrix Element"=-7.093832277304026, "Real Matrix Element"=15.891945503115007}, {"Real Matrix Element"=-7.1975273047975925, "Real Matrix Element"=15.502328165156113}, {"Real Matrix Element"=-7.182524427074781, "Real Matrix Element"=15.511236438640086}, {"Real Matrix Element"=-7.207935486933849, "Real Matrix Element"=15.332406472970602}, {"Real Matrix Element"=-7.33298989800401, "Real Matrix Element"=15.361974821667816}, {"Real Matrix Element"=-7.328927376282974, "Real Matrix Element"=15.254854980372592}, {"Real Matrix Element"=-7.528608407254015, "Real Matrix Element"=15.140521449124785}, {"Real Matrix Element"=-7.429960986327791, "Real Matrix Element"=15.202884434688105}, {"Real Matrix Element"=-7.439687111390317, "Real Matrix Element"=15.187222704892175}, {"Real Matrix Element"=-7.494106574931756, "Real Matrix Element"=15.116468037783175}, {"Real Matrix Element"=-7.658609681188845, "Real Matrix Element"=15.11561548913067}, {"Real Matrix Element"=-7.780691616467418, "Real Matrix Element"=15.015114340322683}, {"Real Matrix Element"=-7.689865899375432, "Real Matrix Element"=14.820414767757919}, {"Real Matrix Element"=-7.6839558626313265, "Real Matrix Element"=14.728556437653335}, {"Real Matrix Element"=-7.674353271257339, "Real Matrix Element"=14.776781700726355}, {"Real Matrix Element"=-7.643006660828978, "Real Matrix Element"=14.602337477627957}, {"Real Matrix Element"=-7.7998980535819715, "Real Matrix Element"=14.660454425022639}, {"Real Matrix Element"=-7.796143189120345, "Real Matrix Element"=14.383243635645066}, {"Real Matrix Element"=-7.896010609138313, "Real Matrix Element"=14.274816700277254}, {"Real Matrix Element"=-7.794318845697075, "Real Matrix Element"=13.877590459671454}, {"Real Matrix Element"=-7.812021682325684, "Real Matrix Element"=13.713272437111833}, {"Real Matrix Element"=-7.960867795050728, "Real Matrix Element"=13.990732187110314}, {"Real Matrix Element"=-7.833106832464487, "Real Matrix Element"=13.738338417965958}, {"Real Matrix Element"=-7.844562335973637, "Real Matrix Element"=13.462479712388951}, {"Real Matrix Element"=-7.903852144185858, "Real Matrix Element"=13.473352592932887}, {"Real Matrix Element"=-8.065304197128675, "Real Matrix Element"=13.4378282790699}, {"Real Matrix Element"=-8.25130421531405, "Real Matrix Element"=13.294317476799502}, {"Real Matrix Element"=-8.132201518823837, "Real Matrix Element"=13.152346655302708}, {"Real Matrix Element"=-8.307641972389263, "Real Matrix Element"=13.069753343116005}, {"Real Matrix Element"=-8.281975155153193, "Real Matrix Element"=12.931463537272961}, {"Real Matrix Element"=-8.395212143221675, "Real Matrix Element"=12.986085595505926}, {"Real Matrix Element"=-8.549968404478252, "Real Matrix Element"=12.88750725470199}, {"Real Matrix Element"=-8.63887497623489, "Real Matrix Element"=12.745704421713429}, {"Real Matrix Element"=-8.70148144976949, "Real Matrix Element"=12.810499180766643}, {"Real Matrix Element"=-8.801189715033782, "Real Matrix Element"=12.647886091897465}, {"Real Matrix Element"=-8.760549637549483, "Real Matrix Element"=12.684756165480414}, {"Real Matrix Element"=-8.819178512849604, "Real Matrix Element"=12.47574552897585}, {"Real Matrix Element"=-8.758401061442301, "Real Matrix Element"=12.414686191520227}, {"Real Matrix Element"=-8.575424262186859, "Real Matrix Element"=12.146483425269366}, {"Real Matrix Element"=-8.700725363003155, "Real Matrix Element"=12.049494787025234}, {"Real Matrix Element"=-8.682606298694578, "Real Matrix Element"=11.817125530124539}, {"Real Matrix Element"=-8.759136906013598, "Real Matrix Element"=11.992582890919932}, {"Real Matrix Element"=-8.790557120752483, "Real Matrix Element"=11.967020986683693}, {"Real Matrix Element"=-8.609528271724056, "Real Matrix Element"=11.33790414314485}, {"Real Matrix Element"=-8.638194940580826, "Real Matrix Element"=11.407154549981817}, {"Real Matrix Element"=-8.641137386256737, "Real Matrix Element"=11.218982127849326}, {"Real Matrix Element"=-8.663693129665127, "Real Matrix Element"=11.050867712968024}, {"Real Matrix Element"=-8.703290506897918, "Real Matrix Element"=11.082585657293471}, {"Real Matrix Element"=-8.69008615702899, "Real Matrix Element"=10.828477546233902}, {"Real Matrix Element"=-8.605893690741777, "Real Matrix Element"=10.74428902897853}, {"Real Matrix Element"=-8.753359287809173, "Real Matrix Element"=10.766216374729575}, {"Real Matrix Element"=-8.568650487142236, "Real Matrix Element"=10.512931821638261}, {"Real Matrix Element"=-8.652105912099065, "Real Matrix Element"=10.478174866524684}, {"Real Matrix Element"=-8.67238018595734, "Real Matrix Element"=10.380024538165646}, {"Real Matrix Element"=-8.742981111745241, "Real Matrix Element"=10.129411412571805}, {"Real Matrix Element"=-8.866337801066775, "Real Matrix Element"=10.321251111430957}, {"Real Matrix Element"=-8.731841140820254, "Real Matrix Element"=10.031371541740604}, {"Real Matrix Element"=-8.678189067233133, "Real Matrix Element"=10.167343164846988}, {"Real Matrix Element"=-8.787382776251448, "Real Matrix Element"=9.981986117345311}, {"Real Matrix Element"=-8.84912298893797, "Real Matrix Element"=10.032702443280312}, {"Real Matrix Element"=-8.716578146854728, "Real Matrix Element"=9.77094097597955}, {"Real Matrix Element"=-8.821996027221923, "Real Matrix Element"=9.800102806068898}, {"Real Matrix Element"=-8.798668501802075, "Real Matrix Element"=9.764654267860463}, {"Real Matrix Element"=-9.032914120121035, "Real Matrix Element"=9.886262572064815}, {"Real Matrix Element"=-9.125709767335515, "Real Matrix Element"=9.83744075757487}, {"Real Matrix Element"=-8.929761113168691, "Real Matrix Element"=9.648573898372744}, {"Real Matrix Element"=-8.901612977946622, "Real Matrix Element"=9.48349899636023}, {"Real Matrix Element"=-9.082858368333525, "Real Matrix Element"=9.348598326792697}, {"Real Matrix Element"=-9.077255830529735, "Real Matrix Element"=9.174825949086237}, {"Real Matrix Element"=-8.881758436323556, "Real Matrix Element"=9.022851290845296}, {"Real Matrix Element"=-8.93685104209657, "Real Matrix Element"=9.00228448634377}, {"Real Matrix Element"=-9.047665947224877, "Real Matrix Element"=9.033215708454264}, {"Real Matrix Element"=-9.04915780797711, "Real Matrix Element"=8.855190790974213}, {"Real Matrix Element"=-9.079687708436742, "Real Matrix Element"=8.810116842805513}, {"Real Matrix Element"=-9.099161938430642, "Real Matrix Element"=8.657626847452509}, {"Real Matrix Element"=-9.092057817438935, "Real Matrix Element"=8.664837954393358}, {"Real Matrix Element"=-8.856686859268846, "Real Matrix Element"=8.399484300901566}, {"Real Matrix Element"=-9.092597179463098, "Real Matrix Element"=8.398883184742466}, {"Real Matrix Element"=-9.031919150621095, "Real Matrix Element"=8.339197379611168}, {"Real Matrix Element"=-8.958738539115553, "Real Matrix Element"=8.288895315966094}, {"Real Matrix Element"=-9.019811997742218, "Real Matrix Element"=8.230157339800666}, {"Real Matrix Element"=-9.037608270025432, "Real Matrix Element"=8.13715591016666}, {"Real Matrix Element"=-9.035184320670723, "Real Matrix Element"=8.106690812873701}, {"Real Matrix Element"=-8.916121215700269, "Real Matrix Element"=8.027745801274195}, {"Real Matrix Element"=-8.992797785277869, "Real Matrix Element"=7.978827035070887}, {"Real Matrix Element"=-8.889006714963893, "Real Matrix Element"=7.816532025042324}, {"Real Matrix Element"=-8.860544251861672, "Real Matrix Element"=7.59316209054098}, {"Real Matrix Element"=-8.751191129977677, "Real Matrix Element"=7.41353510518995}, {"Real Matrix Element"=-8.950258554432823, "Real Matrix Element"=7.479595328765653}, {"Real Matrix Element"=-8.895240151006735, "Real Matrix Element"=7.304170031051378}, {"Real Matrix Element"=-8.756235278325242, "Real Matrix Element"=7.164843003343561}, {"Real Matrix Element"=-8.667257183922025, "Real Matrix Element"=7.10962697662626}, {"Real Matrix Element"=-8.565886871831431, "Real Matrix Element"=6.859618288592279}, {"Real Matrix Element"=-8.682780768470488, "Real Matrix Element"=6.946115819894924}, {"Real Matrix Element"=-8.543654201312327, "Real Matrix Element"=6.619606235803255}, {"Real Matrix Element"=-8.450996544705575, "Real Matrix Element"=6.4136113633896725}, {"Real Matrix Element"=-8.384154051613333, "Real Matrix Element"=6.339659582273761}, {"Real Matrix Element"=-8.338018650876093, "Real Matrix Element"=6.313415947162766}, {"Real Matrix Element"=-8.420450500357887, "Real Matrix Element"=6.267945919506862}, {"Real Matrix Element"=-8.287126479576605, "Real Matrix Element"=6.202849699041565}, {"Real Matrix Element"=-8.209048617838938, "Real Matrix Element"=6.07290514954744}, {"Real Matrix Element"=-8.27620356712854, "Real Matrix Element"=5.991657726331528}, {"Real Matrix Element"=-8.24962423308571, "Real Matrix Element"=6.005431098328958}, {"Real Matrix Element"=-8.106936551806955, "Real Matrix Element"=5.872453285838931}, {"Real Matrix Element"=-8.126437125967517, "Real Matrix Element"=5.73746638328293}, {"Real Matrix Element"=-8.05878515700632, "Real Matrix Element"=5.571855539530804}, {"Real Matrix Element"=-7.99717428292569, "Real Matrix Element"=5.490472668392403}, {"Real Matrix Element"=-7.834056869284986, "Real Matrix Element"=5.334441588531236}, {"Real Matrix Element"=-7.957990734548831, "Real Matrix Element"=5.36745672283707}, {"Real Matrix Element"=-8.011163777739563, "Real Matrix Element"=5.391305866310304}, {"Real Matrix Element"=-8.198237974770288, "Real Matrix Element"=5.307031746703785}, {"Real Matrix Element"=-8.11519143124797, "Real Matrix Element"=5.176483117437406}, {"Real Matrix Element"=-8.078240913300272, "Real Matrix Element"=5.045701100074011}, {"Real Matrix Element"=-8.042962648083812, "Real Matrix Element"=4.976982321349185}, {"Real Matrix Element"=-7.968617223184104, "Real Matrix Element"=4.891771591630298}, {"Real Matrix Element"=-8.046054429239181, "Real Matrix Element"=4.838908404077888}, {"Real Matrix Element"=-7.837473601929452, "Real Matrix Element"=4.694456847852686}, {"Real Matrix Element"=-7.982315428969225, "Real Matrix Element"=4.6499097700915195}, {"Real Matrix Element"=-8.071437676481208, "Real Matrix Element"=4.618344756341493}, {"Real Matrix Element"=-7.99110782390612, "Real Matrix Element"=4.551447867902977}, {"Real Matrix Element"=-7.822974414448834, "Real Matrix Element"=4.414409561558992}, {"Real Matrix Element"=-7.765764926929625, "Real Matrix Element"=4.332609439207336}, {"Real Matrix Element"=-7.392186683915942, "Real Matrix Element"=4.173316970762073}, {"Real Matrix Element"=-7.318837238756243, "Real Matrix Element"=4.128140214911549}, {"Real Matrix Element"=-7.340263855557005, "Real Matrix Element"=4.087917652523148}, {"Real Matrix Element"=-7.328217602355016, "Real Matrix Element"=3.9830675418004993}, {"Real Matrix Element"=-7.3114433482862395, "Real Matrix Element"=3.910935660320266}, {"Real Matrix Element"=-7.101677023585898, "Real Matrix Element"=3.8449573030442545}, {"Real Matrix Element"=-7.052394341073253, "Real Matrix Element"=3.876875266758225}, {"Real Matrix Element"=-7.100121365855529, "Real Matrix Element"=3.7806507388637294}, {"Real Matrix Element"=-6.984070904052292, "Real Matrix Element"=3.700348976567538}, {"Real Matrix Element"=-6.762816779642208, "Real Matrix Element"=3.618458299235416}, {"Real Matrix Element"=-6.704327102063188, "Real Matrix Element"=3.5065248377100615}, {"Real Matrix Element"=-6.692085740303761, "Real Matrix Element"=3.4299142199098878}, {"Real Matrix Element"=-6.680619695265483, "Real Matrix Element"=3.4195419055384635}, {"Real Matrix Element"=-6.465263550943983, "Real Matrix Element"=3.2057806040543606}, {"Real Matrix Element"=-6.472383252334107, "Real Matrix Element"=3.225228127857129}, {"Real Matrix Element"=-6.487720580063696, "Real Matrix Element"=3.137590057615895}, {"Real Matrix Element"=-6.59383142318151, "Real Matrix Element"=3.14076946652414}, {"Real Matrix Element"=-6.352526013599931, "Real Matrix Element"=3.09853402629643}, {"Real Matrix Element"=-6.268176611782154, "Real Matrix Element"=3.0475296719604743}, {"Real Matrix Element"=-6.237254475906482, "Real Matrix Element"=2.9079536918139914}, {"Real Matrix Element"=-6.198064502692333, "Real Matrix Element"=2.8840355107603464}, {"Real Matrix Element"=-6.075402830674424, "Real Matrix Element"=2.8107407970942586}, {"Real Matrix Element"=-6.036856663425191, "Real Matrix Element"=2.6971665730623027}, {"Real Matrix Element"=-5.80596068890998, "Real Matrix Element"=2.5128009487895246}, {"Real Matrix Element"=-5.614050473024162, "Real Matrix Element"=2.397268520107794}, {"Real Matrix Element"=-5.431412121141701, "Real Matrix Element"=2.290130825589646}, {"Real Matrix Element"=-5.312226935969562, "Real Matrix Element"=2.200117077120997}, {"Real Matrix Element"=-5.499293586228612, "Real Matrix Element"=2.209183423387926}, {"Real Matrix Element"=-5.5207867129204695, "Real Matrix Element"=2.191104982830947}, {"Real Matrix Element"=-5.277183672098678, "Real Matrix Element"=1.9153771348763649}, {"Real Matrix Element"=-5.144720104287786, "Real Matrix Element"=1.878571709636136}, {"Real Matrix Element"=-5.026296037877472, "Real Matrix Element"=1.9803031663736779}, {"Real Matrix Element"=-4.869338160763627, "Real Matrix Element"=1.9297875037562844}, {"Real Matrix Element"=-4.954614239442981, "Real Matrix Element"=1.996588497004235}, {"Real Matrix Element"=-4.978570218106093, "Real Matrix Element"=1.8722461736023692}, {"Real Matrix Element"=-4.836193331797336, "Real Matrix Element"=1.6927380310409337}, {"Real Matrix Element"=-4.628985172773662, "Real Matrix Element"=1.666624641876256}, {"Real Matrix Element"=-4.707595186570373, "Real Matrix Element"=1.5633556880670867}, {"Real Matrix Element"=-4.698208046125662, "Real Matrix Element"=1.461733354581974}, {"Real Matrix Element"=-4.451653414742413, "Real Matrix Element"=1.256967022617457}, {"Real Matrix Element"=-4.362427480743445, "Real Matrix Element"=1.4129313264260477}, {"Real Matrix Element"=-4.306999790770671, "Real Matrix Element"=1.614739578563848}, {"Real Matrix Element"=-4.134231299271714, "Real Matrix Element"=1.3962723299039643}, {"Real Matrix Element"=-3.9838119813358173, "Real Matrix Element"=1.1150503511913468}, {"Real Matrix Element"=-3.9470447384943657, "Real Matrix Element"=1.036936065335949}, {"Real Matrix Element"=-3.9321062696173152, "Real Matrix Element"=1.1158775870015931}, {"Real Matrix Element"=-3.838335468026536, "Real Matrix Element"=0.9514923585548307}, {"Real Matrix Element"=-3.941808442732729, "Real Matrix Element"=1.00491308005979}, {"Real Matrix Element"=-3.760361137177643, "Real Matrix Element"=0.9631345159204427}, {"Real Matrix Element"=-3.582759781020441, "Real Matrix Element"=0.8072515956570558}, {"Real Matrix Element"=-3.49859229685737, "Real Matrix Element"=1.1310165612185705}, {"Real Matrix Element"=-3.506713289435365, "Real Matrix Element"=1.1081262983655913}, {"Real Matrix Element"=-3.321965665082041, "Real Matrix Element"=0.8092142941290138}, {"Real Matrix Element"=-3.3234142760900456, "Real Matrix Element"=0.8770551389941437}, {"Real Matrix Element"=-3.1979676652667925, "Real Matrix Element"=0.7349697794228334}, {"Real Matrix Element"=-3.150222191917882, "Real Matrix Element"=0.7254689864646328}, {"Real Matrix Element"=-3.155463379052734, "Real Matrix Element"=0.5871854694774729}, {"Real Matrix Element"=-3.14183031975483, "Real Matrix Element"=0.727272006464919}, {"Real Matrix Element"=-3.1684840942771473, "Real Matrix Element"=0.6645293590442733}, {"Real Matrix Element"=-3.207180086321945, "Real Matrix Element"=0.7429020885628569}, {"Real Matrix Element"=-2.989217242874688, "Real Matrix Element"=0.6834589744296153}, {"Real Matrix Element"=-2.784861696131446, "Real Matrix Element"=0.6664529896338737}, {"Real Matrix Element"=-2.72039229756656, "Real Matrix Element"=0.6499874759588433}, {"Real Matrix Element"=-2.5753874487380886, "Real Matrix Element"=0.6570032146599306}, {"Real Matrix Element"=-2.60691301578771, "Real Matrix Element"=0.5057428880498372}, {"Real Matrix Element"=-2.3701483218237107, "Real Matrix Element"=0.37133854987786497}, {"Real Matrix Element"=-2.2217305142236983, "Real Matrix Element"=0.2603991344651112}, {"Real Matrix Element"=-2.0365139106641506, "Real Matrix Element"=0.31562919240471454}, {"Real Matrix Element"=-1.712238914395592, "Real Matrix Element"=0.15685587313609622}, {"Real Matrix Element"=-1.539802948923146, "Real Matrix Element"=0.05716918717711794}, {"Real Matrix Element"=-1.3898872474522492, "Real Matrix Element"=0.1700604853303716}, {"Real Matrix Element"=-1.5470953519087607, "Real Matrix Element"=0.26710597289884347}, {"Real Matrix Element"=-1.4290755329599014, "Real Matrix Element"=0.2747295667241359}, {"Real Matrix Element"=-1.4120900092480195, "Real Matrix Element"=0.39672992116214273}, {"Real Matrix Element"=-1.2605330756073947, "Real Matrix Element"=0.3520162244733124}, {"Real Matrix Element"=-1.3829333087515332, "Real Matrix Element"=0.32898526406336964}, {"Real Matrix Element"=-1.3316704669052946, "Real Matrix Element"=0.2629322754779213}, {"Real Matrix Element"=-1.1239286490963347, "Real Matrix Element"=0.20290470454836962}, {"Real Matrix Element"=-0.9179952725136848, "Real Matrix Element"=0.23434088588916976}, {"Real Matrix Element"=-0.9013843175909172, "Real Matrix Element"=0.14275606646094982}, {"Real Matrix Element"=-0.9587211751404034, "Real Matrix Element"=0.16860740211487174}, {"Real Matrix Element"=-0.6665387442193272, "Real Matrix Element"=0.18405216435410812}, {"Real Matrix Element"=-0.6313729800059624, "Real Matrix Element"=0.12091357383542575}, {"Real Matrix Element"=-0.5249302526351416, "Real Matrix Element"=0.1475249524804513}, {"Real Matrix Element"=-0.5520182546082153, "Real Matrix Element"=0.14881248675596917}, {"Real Matrix Element"=-0.43662459027116474, "Real Matrix Element"=0.12186296094992549}, {"Real Matrix Element"=-0.3586199916459565, "Real Matrix Element"=0.19306995029431157}, {"Real Matrix Element"=-0.1955113688479492, "Real Matrix Element"=0.1685923104105771}, {"Real Matrix Element"=-0.15068540035599035, "Real Matrix Element"=0.027884099756623343}, {"Real Matrix Element"=-0.014072639199940382, "Real Matrix Element"=0.0445501270189739}, {"Real Matrix Element"=0.0140964514810892, "Real Matrix Element"=-0.05265633240063431}, {"Real Matrix Element"=0.29253989613065284, "Real Matrix Element"=0.11318694523456577}, {"Real Matrix Element"=0.2957986714486853, "Real Matrix Element"=0.06772591550252523}, {"Real Matrix Element"=0.4102737687218699, "Real Matrix Element"=0.05195973450704134}, {"Real Matrix Element"=0.4937606423809629, "Real Matrix Element"=0.027510625323047176}, {"Real Matrix Element"=0.5941213811270711, "Real Matrix Element"=-0.10321021889958268}, {"Real Matrix Element"=0.7885420678132599, "Real Matrix Element"=0.0008001391690772436}, {"Real Matrix Element"=0.8940221412347962, "Real Matrix Element"=0.18210073568350113}, {"Real Matrix Element"=0.7971892216426472, "Real Matrix Element"=0.08339778085587815}, {"Real Matrix Element"=0.8587265176469272, "Real Matrix Element"=0.28595243591621816}, {"Real Matrix Element"=0.9818281893652788, "Real Matrix Element"=0.3360830919797222}, {"Real Matrix Element"=0.9787217667187763, "Real Matrix Element"=0.22525972203946998}, {"Real Matrix Element"=1.192520629498687, "Real Matrix Element"=0.16384094743949823}, {"Real Matrix Element"=1.1707441498879023, "Real Matrix Element"=-0.022503934108357743}, {"Real Matrix Element"=1.4536354921122214, "Real Matrix Element"=0.19612984453441684}, {"Real Matrix Element"=1.6150783600977054, "Real Matrix Element"=0.1381861382458947}, {"Real Matrix Element"=1.6880043965602847, "Real Matrix Element"=0.1135933674319885}, {"Real Matrix Element"=1.6543416784839498, "Real Matrix Element"=-0.01251633047330937}, {"Real Matrix Element"=1.8632431996485213, "Real Matrix Element"=0.0930801047702364}, {"Real Matrix Element"=1.8782766402359496, "Real Matrix Element"=0.0016500730945784997}, {"Real Matrix Element"=1.919213366246777, "Real Matrix Element"=0.36481996136512207}, {"Real Matrix Element"=2.0927008991427196, "Real Matrix Element"=0.24853219079718214}, {"Real Matrix Element"=2.2344471216104798, "Real Matrix Element"=0.7276812180294431}, {"Real Matrix Element"=2.153925623344385, "Real Matrix Element"=0.503210981517721}, {"Real Matrix Element"=2.3212540059532594, "Real Matrix Element"=0.6315284221251907}, {"Real Matrix Element"=2.499887987302666, "Real Matrix Element"=0.4886359553863617}, {"Real Matrix Element"=2.546178503260841, "Real Matrix Element"=0.45944144574192963}, {"Real Matrix Element"=2.740631846989087, "Real Matrix Element"=0.6248814812624144}, {"Real Matrix Element"=2.8641018952940493, "Real Matrix Element"=0.477385741138032}, {"Real Matrix Element"=2.9970995327310503, "Real Matrix Element"=0.46097136947394596}, {"Real Matrix Element"=3.087042429525038, "Real Matrix Element"=0.4252262305488586}, {"Real Matrix Element"=3.3970193535349305, "Real Matrix Element"=0.5302016042441106}, {"Real Matrix Element"=3.450291347853067, "Real Matrix Element"=0.358042984382586}, {"Real Matrix Element"=3.5624895119361337, "Real Matrix Element"=0.5988259437853825}, {"Real Matrix Element"=3.4925657052937362, "Real Matrix Element"=0.5036466442668455}, {"Real Matrix Element"=3.5322645032021973, "Real Matrix Element"=0.3801874703158487}, {"Real Matrix Element"=3.7500635888656046, "Real Matrix Element"=0.5306387024862097}, {"Real Matrix Element"=3.826603864602047, "Real Matrix Element"=0.6532091378147464}, {"Real Matrix Element"=3.8859051322897837, "Real Matrix Element"=0.654554859539244}, {"Real Matrix Element"=3.9284668085881824, "Real Matrix Element"=0.7719980756737361}, {"Real Matrix Element"=3.9691072218697645, "Real Matrix Element"=0.9249980927869579}, {"Real Matrix Element"=3.9819097030382964, "Real Matrix Element"=0.8230846331613826}, {"Real Matrix Element"=4.084602345488705, "Real Matrix Element"=1.0733076594103963}, {"Real Matrix Element"=4.229729856487897, "Real Matrix Element"=1.2158173107870591}, {"Real Matrix Element"=4.264579852953784, "Real Matrix Element"=0.9626827324759271}, {"Real Matrix Element"=4.375981658053042, "Real Matrix Element"=0.9548916115279671}, {"Real Matrix Element"=4.498539751617972, "Real Matrix Element"=0.9104268248633317}, {"Real Matrix Element"=4.645499995159645, "Real Matrix Element"=1.2315824683300218}, {"Real Matrix Element"=4.655201779537502, "Real Matrix Element"=1.149665120140367}, {"Real Matrix Element"=4.8550069716901785, "Real Matrix Element"=1.48235144598572}, {"Real Matrix Element"=4.89101279913061, "Real Matrix Element"=1.4399024587185072}, {"Real Matrix Element"=4.959073684146854, "Real Matrix Element"=1.5543803948460921}, {"Real Matrix Element"=5.065215215406938, "Real Matrix Element"=1.4182095357861964}, {"Real Matrix Element"=5.158262533094799, "Real Matrix Element"=1.4930621554095194}, {"Real Matrix Element"=5.107690065970033, "Real Matrix Element"=1.2993942567847687}, {"Real Matrix Element"=5.203408899779102, "Real Matrix Element"=1.42214678739009}, {"Real Matrix Element"=5.28156448819088, "Real Matrix Element"=1.4995110604554966}, {"Real Matrix Element"=5.433995620604159, "Real Matrix Element"=1.7608811125565222}, {"Real Matrix Element"=5.576282878928627, "Real Matrix Element"=1.7173771552293713}, {"Real Matrix Element"=5.604615214121901, "Real Matrix Element"=1.5784172696233754}, {"Real Matrix Element"=5.674182512998902, "Real Matrix Element"=1.4479333042471705}, {"Real Matrix Element"=5.715678421738508, "Real Matrix Element"=1.5952771544117614}, {"Real Matrix Element"=5.764619286468771, "Real Matrix Element"=1.6092314961597953}, {"Real Matrix Element"=5.713751758538035, "Real Matrix Element"=1.7768871591908564}, {"Real Matrix Element"=5.828825105542899, "Real Matrix Element"=1.9883627698781245}, {"Real Matrix Element"=5.952845571834138, "Real Matrix Element"=2.130584930909256}, {"Real Matrix Element"=6.084570550882689, "Real Matrix Element"=2.2464460780195914}, {"Real Matrix Element"=6.242067279344121, "Real Matrix Element"=2.260309388477042}, {"Real Matrix Element"=6.336333497358721, "Real Matrix Element"=2.4026614243084707}, {"Real Matrix Element"=6.454790428146973, "Real Matrix Element"=2.772785426702312}, {"Real Matrix Element"=6.564281798398709, "Real Matrix Element"=2.5184633804810628}, {"Real Matrix Element"=6.642433668000771, "Real Matrix Element"=2.820339117761022}, {"Real Matrix Element"=6.676596161154426, "Real Matrix Element"=2.848919266755198}, {"Real Matrix Element"=6.600076762728575, "Real Matrix Element"=2.7688385347843147}, {"Real Matrix Element"=6.650355716349817, "Real Matrix Element"=2.8569445004289307}, {"Real Matrix Element"=6.719159718608088, "Real Matrix Element"=2.814493657816228}, {"Real Matrix Element"=6.790222751336357, "Real Matrix Element"=2.880934240199125}, {"Real Matrix Element"=6.81212242682845, "Real Matrix Element"=2.8631411073303417}, {"Real Matrix Element"=6.935272518635239, "Real Matrix Element"=2.8554675795871343}, {"Real Matrix Element"=7.018199383489161, "Real Matrix Element"=3.047360864392008}, {"Real Matrix Element"=7.172900143331294, "Real Matrix Element"=3.3438822276954987}, {"Real Matrix Element"=7.211260578898494, "Real Matrix Element"=3.370889282343841}, {"Real Matrix Element"=7.2744143729126804, "Real Matrix Element"=3.3781749636375475}, {"Real Matrix Element"=7.277876872078054, "Real Matrix Element"=3.1017114603181306}, {"Real Matrix Element"=7.3690848993175155, "Real Matrix Element"=3.3839863568402153}, {"Real Matrix Element"=7.4465851853979625, "Real Matrix Element"=3.4559580024255068}, {"Real Matrix Element"=7.481618169352075, "Real Matrix Element"=3.699250659311195}, {"Real Matrix Element"=7.4806247927607075, "Real Matrix Element"=3.4889832104079477}, {"Real Matrix Element"=7.505953634628771, "Real Matrix Element"=3.6357913226402014}, {"Real Matrix Element"=7.581045186782927, "Real Matrix Element"=3.762810704744466}, {"Real Matrix Element"=7.661935457461418, "Real Matrix Element"=4.073208463428093}, {"Real Matrix Element"=7.706737316425872, "Real Matrix Element"=4.07519958594739}, {"Real Matrix Element"=7.809153451123742, "Real Matrix Element"=3.96902445179542}, {"Real Matrix Element"=7.893195247497763, "Real Matrix Element"=4.140288809915808}, {"Real Matrix Element"=7.975479254173516, "Real Matrix Element"=4.182560349146938}, {"Real Matrix Element"=8.063148918359792, "Real Matrix Element"=4.288008114123124}, {"Real Matrix Element"=8.066979863978807, "Real Matrix Element"=4.167447635229871}, {"Real Matrix Element"=8.188260497362483, "Real Matrix Element"=4.660515833513064}, {"Real Matrix Element"=8.20222706696863, "Real Matrix Element"=4.434702304865374}, {"Real Matrix Element"=8.220491642723179, "Real Matrix Element"=4.366175129442491}, {"Real Matrix Element"=8.276938547234474, "Real Matrix Element"=4.668977989678396}, {"Real Matrix Element"=8.28688729038884, "Real Matrix Element"=4.7057034597850755}, {"Real Matrix Element"=8.375279508082821, "Real Matrix Element"=4.946257549376104}, {"Real Matrix Element"=8.436496442024957, "Real Matrix Element"=4.794173250118568}, {"Real Matrix Element"=8.468596464416391, "Real Matrix Element"=4.952029900024416}, {"Real Matrix Element"=8.50777513607058, "Real Matrix Element"=5.111400231475035}, {"Real Matrix Element"=8.51383639152451, "Real Matrix Element"=5.129875998253703}, {"Real Matrix Element"=8.544933089061605, "Real Matrix Element"=5.187070945963629}, {"Real Matrix Element"=8.576173249213609, "Real Matrix Element"=5.222834915893765}, {"Real Matrix Element"=8.648837542398176, "Real Matrix Element"=5.450047721551394}, {"Real Matrix Element"=8.683267688627843, "Real Matrix Element"=5.656715059197657}, {"Real Matrix Element"=8.728938667050134, "Real Matrix Element"=5.4800139419605625}, {"Real Matrix Element"=8.738601276450066, "Real Matrix Element"=5.711911130031412}, {"Real Matrix Element"=8.736606155471662, "Real Matrix Element"=5.799453103629842}, {"Real Matrix Element"=8.753146375370235, "Real Matrix Element"=5.807204183384298}, {"Real Matrix Element"=8.7961132760856, "Real Matrix Element"=5.898361095939456}, {"Real Matrix Element"=8.796184769912637, "Real Matrix Element"=6.284828342190563}, {"Real Matrix Element"=8.795833510588919, "Real Matrix Element"=6.357381352915778}, {"Real Matrix Element"=8.863461292240862, "Real Matrix Element"=6.2983200806584705}, {"Real Matrix Element"=8.789048028598557, "Real Matrix Element"=6.683160492822993}, {"Real Matrix Element"=8.744328967210748, "Real Matrix Element"=6.546702346156461}, {"Real Matrix Element"=8.804985124952209, "Real Matrix Element"=6.742157299893477}, {"Real Matrix Element"=8.817617425153536, "Real Matrix Element"=6.94838395972071}, {"Real Matrix Element"=8.877809071294111, "Real Matrix Element"=6.804957882077066}, {"Real Matrix Element"=9.015472739959131, "Real Matrix Element"=6.8528966849342146}, {"Real Matrix Element"=8.917650836431866, "Real Matrix Element"=6.823098915577198}, {"Real Matrix Element"=8.965790956817823, "Real Matrix Element"=6.646961555630436}, {"Real Matrix Element"=9.016929345413288, "Real Matrix Element"=6.970150745857504}, {"Real Matrix Element"=8.935932086781415, "Real Matrix Element"=7.253574851432868}, {"Real Matrix Element"=8.989702942589208, "Real Matrix Element"=7.4141289110833695}, {"Real Matrix Element"=9.030171499231628, "Real Matrix Element"=7.6489125001438145}, {"Real Matrix Element"=9.098493193678715, "Real Matrix Element"=7.496958139727607}, {"Real Matrix Element"=9.212000891719494, "Real Matrix Element"=8.139102695162649}, {"Real Matrix Element"=9.185439067035189, "Real Matrix Element"=7.994120048757125}, {"Real Matrix Element"=9.304315863405725, "Real Matrix Element"=7.987690613728993}, {"Real Matrix Element"=9.248578409811813, "Real Matrix Element"=8.04930103371877}, {"Real Matrix Element"=9.2594557119449, "Real Matrix Element"=8.134764543642031}, {"Real Matrix Element"=9.294510660473366, "Real Matrix Element"=8.228692663040377}, {"Real Matrix Element"=9.24698497350918, "Real Matrix Element"=8.360366814156816}, {"Real Matrix Element"=9.334172558650973, "Real Matrix Element"=8.120657127798856}, {"Real Matrix Element"=9.336630059093677, "Real Matrix Element"=8.47814408193799}, {"Real Matrix Element"=9.48591270597527, "Real Matrix Element"=8.405085437579537}, {"Real Matrix Element"=9.482430003509268, "Real Matrix Element"=8.697611008870739}, {"Real Matrix Element"=9.618523615557606, "Real Matrix Element"=8.960379951570816}, {"Real Matrix Element"=9.534454310299845, "Real Matrix Element"=8.693461410230848}, {"Real Matrix Element"=9.633569889730083, "Real Matrix Element"=8.866551006401957}, {"Real Matrix Element"=9.626844690432335, "Real Matrix Element"=8.627305461178523}, {"Real Matrix Element"=9.677790695958281, "Real Matrix Element"=8.803170265476313}, {"Real Matrix Element"=9.606473286859647, "Real Matrix Element"=9.253933651724216}, {"Real Matrix Element"=9.538015804663228, "Real Matrix Element"=9.356492793481983}, {"Real Matrix Element"=9.563671787843006, "Real Matrix Element"=9.494913550656449}, {"Real Matrix Element"=9.628585841108327, "Real Matrix Element"=9.413560685978942}, {"Real Matrix Element"=9.617107968092691, "Real Matrix Element"=9.678264660237462}, {"Real Matrix Element"=9.710321515787465, "Real Matrix Element"=9.665447697127194}, {"Real Matrix Element"=9.627305763215459, "Real Matrix Element"=9.89922218674036}, {"Real Matrix Element"=9.671037271026659, "Real Matrix Element"=10.028256531366031}, {"Real Matrix Element"=9.65617809055663, "Real Matrix Element"=9.9771186438688}, {"Real Matrix Element"=9.58781063701936, "Real Matrix Element"=10.091330427951911}, {"Real Matrix Element"=9.574340588680753, "Real Matrix Element"=10.314518180973515}, {"Real Matrix Element"=9.657876639809686, "Real Matrix Element"=10.245940142452106}, {"Real Matrix Element"=9.712219823008658, "Real Matrix Element"=10.457270375776833}, {"Real Matrix Element"=9.778111283284183, "Real Matrix Element"=10.240074278002998}, {"Real Matrix Element"=9.692055334867645, "Real Matrix Element"=10.362131345682124}, {"Real Matrix Element"=9.65826910396971, "Real Matrix Element"=10.575665739576207}, {"Real Matrix Element"=9.67991510341283, "Real Matrix Element"=11.018280761318975}, {"Real Matrix Element"=9.738846061358563, "Real Matrix Element"=11.305815127287966}, {"Real Matrix Element"=9.81168508663788, "Real Matrix Element"=11.390898157872426}, {"Real Matrix Element"=9.737341209192403, "Real Matrix Element"=11.175289030868408}, {"Real Matrix Element"=9.565264375392024, "Real Matrix Element"=11.171150895223475}, {"Real Matrix Element"=9.525215017729785, "Real Matrix Element"=11.261984193687422}, {"Real Matrix Element"=9.567832261621247, "Real Matrix Element"=11.242298063198362}, {"Real Matrix Element"=9.5148933421027, "Real Matrix Element"=11.489318566668288}, {"Real Matrix Element"=9.53137850752679, "Real Matrix Element"=11.49969572327409}, {"Real Matrix Element"=9.600241736642785, "Real Matrix Element"=11.541349816860983}, {"Real Matrix Element"=9.454851031579988, "Real Matrix Element"=11.7350678569986}, {"Real Matrix Element"=9.43836129949595, "Real Matrix Element"=12.065956351042413}, {"Real Matrix Element"=9.477047763630596, "Real Matrix Element"=12.16137907941765}, {"Real Matrix Element"=9.390560590400609, "Real Matrix Element"=12.47846991402048}, {"Real Matrix Element"=9.399919926072018, "Real Matrix Element"=12.34006450721673}, {"Real Matrix Element"=9.192445850795497, "Real Matrix Element"=12.231455654991874}, {"Real Matrix Element"=9.176227466609987, "Real Matrix Element"=12.504195270787688}, {"Real Matrix Element"=9.073879514557195, "Real Matrix Element"=12.655191408884775}, {"Real Matrix Element"=9.121351195994071, "Real Matrix Element"=12.47386795379324}, {"Real Matrix Element"=8.993631986221223, "Real Matrix Element"=12.592093158874677}, {"Real Matrix Element"=9.012735091843464, "Real Matrix Element"=12.775779659071967}, {"Real Matrix Element"=9.00180712138036, "Real Matrix Element"=12.818204428284915}, {"Real Matrix Element"=8.990470118368922, "Real Matrix Element"=12.947785187673173}, {"Real Matrix Element"=9.125147220362354, "Real Matrix Element"=13.050994248834588}, {"Real Matrix Element"=9.14159234216814, "Real Matrix Element"=13.019348227037023}, {"Real Matrix Element"=9.009737404070849, "Real Matrix Element"=13.038290827430197}, {"Real Matrix Element"=9.032272966041905, "Real Matrix Element"=13.127864772081217}, {"Real Matrix Element"=9.24020343356265, "Real Matrix Element"=13.163958415200236}, {"Real Matrix Element"=9.285742776803671, "Real Matrix Element"=13.163571808040075}, {"Real Matrix Element"=9.263035118488439, "Real Matrix Element"=13.236031499265717}, {"Real Matrix Element"=9.192470065370944, "Real Matrix Element"=13.291092875227063}, {"Real Matrix Element"=9.101007935119457, "Real Matrix Element"=13.359789182306985}, {"Real Matrix Element"=9.056608320076691, "Real Matrix Element"=13.47056326911728}, {"Real Matrix Element"=8.922508275980809, "Real Matrix Element"=13.530430310731406}, {"Real Matrix Element"=8.730882491998264, "Real Matrix Element"=13.55347533419244}, {"Real Matrix Element"=8.844530276175004, "Real Matrix Element"=13.711330316770722}, {"Real Matrix Element"=8.798323765914786, "Real Matrix Element"=13.737931927887901}, {"Real Matrix Element"=8.966527762183526, "Real Matrix Element"=13.690102961244818}, {"Real Matrix Element"=8.816279352791781, "Real Matrix Element"=13.93806636972295}, {"Real Matrix Element"=8.95041187180969, "Real Matrix Element"=13.939532920476536}, {"Real Matrix Element"=8.786597032264654, "Real Matrix Element"=13.986117184117356}, {"Real Matrix Element"=8.826236869333982, "Real Matrix Element"=13.890362489522682}, {"Real Matrix Element"=8.653800046739653, "Real Matrix Element"=14.327362761353301}, {"Real Matrix Element"=8.534162478114865, "Real Matrix Element"=14.591822151315192}, {"Real Matrix Element"=8.389247510073552, "Real Matrix Element"=14.521479268236119}, {"Real Matrix Element"=8.349974489069114, "Real Matrix Element"=14.676496230349011}, {"Real Matrix Element"=8.245096954175727, "Real Matrix Element"=15.063041314254205}, {"Real Matrix Element"=8.227031430900608, "Real Matrix Element"=15.0706783562461}, {"Real Matrix Element"=8.092742401727733, "Real Matrix Element"=15.298326642731132}, {"Real Matrix Element"=8.105058724715084, "Real Matrix Element"=15.069915302186676}, {"Real Matrix Element"=7.976293035029383, "Real Matrix Element"=15.151052197619288}, {"Real Matrix Element"=7.8700751770202135, "Real Matrix Element"=15.359081852987703}, {"Real Matrix Element"=7.703989021642525, "Real Matrix Element"=15.49845710481287}, {"Real Matrix Element"=7.682484307430085, "Real Matrix Element"=15.6128108862719}, {"Real Matrix Element"=7.769217262753844, "Real Matrix Element"=15.544296152607}, {"Real Matrix Element"=7.493352676497696, "Real Matrix Element"=15.657053432509048}, {"Real Matrix Element"=7.395637062279723, "Real Matrix Element"=15.704478807902253}, {"Real Matrix Element"=7.413659972341027, "Real Matrix Element"=15.77142973811154}, {"Real Matrix Element"=7.339240588164442, "Real Matrix Element"=15.791945076267629}, {"Real Matrix Element"=7.3148830770805775, "Real Matrix Element"=15.787944949502267}, {"Real Matrix Element"=7.234636424684882, "Real Matrix Element"=15.85934446890968}, {"Real Matrix Element"=7.150944802043242, "Real Matrix Element"=16.070939596459}, {"Real Matrix Element"=7.126337906933936, "Real Matrix Element"=16.02661212794691}, {"Real Matrix Element"=7.074043893194475, "Real Matrix Element"=16.168313340432125}, {"Real Matrix Element"=6.992286480347396, "Real Matrix Element"=16.252032792649807}, {"Real Matrix Element"=6.700655268345445, "Real Matrix Element"=16.322458249853312}, {"Real Matrix Element"=6.5624219924383675, "Real Matrix Element"=16.484049188302585}, {"Real Matrix Element"=6.474935768439322, "Real Matrix Element"=16.3590108036151}, {"Real Matrix Element"=6.432579293814547, "Real Matrix Element"=16.42391395401335}, {"Real Matrix Element"=6.4858480214877625, "Real Matrix Element"=16.38695301375314}, {"Real Matrix Element"=6.528114276198872, "Real Matrix Element"=16.548542036931103}, {"Real Matrix Element"=6.277859205199329, "Real Matrix Element"=16.647589737686108}, {"Real Matrix Element"=6.1460489690984685, "Real Matrix Element"=16.77143950169177}, {"Real Matrix Element"=6.132057515930932, "Real Matrix Element"=16.722858940487697}, {"Real Matrix Element"=6.047154581005624, "Real Matrix Element"=16.76455566916103}, {"Real Matrix Element"=5.996975872597279, "Real Matrix Element"=16.779334739131073}, {"Real Matrix Element"=6.036772395210784, "Real Matrix Element"=17.067101521668057}, {"Real Matrix Element"=6.183764158495983, "Real Matrix Element"=17.241318757569367}, {"Real Matrix Element"=6.125383668871652, "Real Matrix Element"=17.328957521553576}, {"Real Matrix Element"=6.1553506290652455, "Real Matrix Element"=17.145464008814407}, {"Real Matrix Element"=5.992906433974249, "Real Matrix Element"=17.349090401120193}, {"Real Matrix Element"=5.920809757517333, "Real Matrix Element"=17.42738282134887}, {"Real Matrix Element"=5.842584392742744, "Real Matrix Element"=17.332459560303388}, {"Real Matrix Element"=5.951069923348571, "Real Matrix Element"=17.549594098785153}, {"Real Matrix Element"=5.78555861111635, "Real Matrix Element"=17.774181612103323}, {"Real Matrix Element"=5.7367788544060705, "Real Matrix Element"=17.8722105971215}, {"Real Matrix Element"=5.657459679046568, "Real Matrix Element"=17.784665873066952}, {"Real Matrix Element"=5.668305176903491, "Real Matrix Element"=17.860040738461745}, {"Real Matrix Element"=5.552336409784915, "Real Matrix Element"=17.993237943567635}, {"Real Matrix Element"=5.4729881568126855, "Real Matrix Element"=17.95085082340476}, {"Real Matrix Element"=5.412415684934573, "Real Matrix Element"=17.823060592550924}, {"Real Matrix Element"=5.154016060093928, "Real Matrix Element"=17.90328884178995}, {"Real Matrix Element"=4.935444778618575, "Real Matrix Element"=18.07318368906534}, {"Real Matrix Element"=4.974059232066028, "Real Matrix Element"=17.972807940639644}, {"Real Matrix Element"=4.858031010536886, "Real Matrix Element"=18.206977636771665}, {"Real Matrix Element"=4.832198921624965, "Real Matrix Element"=18.331418004108837}, {"Real Matrix Element"=4.7513173576583565, "Real Matrix Element"=18.360676798179554}, {"Real Matrix Element"=4.709967877119229, "Real Matrix Element"=18.53287157446633}, {"Real Matrix Element"=4.535326967644368, "Real Matrix Element"=18.7278671466388}, {"Real Matrix Element"=4.440559417964701, "Real Matrix Element"=18.79648649911499}, {"Real Matrix Element"=4.301848749637914, "Real Matrix Element"=18.96929326418142}, {"Real Matrix Element"=4.212660268315994, "Real Matrix Element"=18.72717420641894}, {"Real Matrix Element"=4.178708400945012, "Real Matrix Element"=18.786746921157746}, {"Real Matrix Element"=4.097214018095873, "Real Matrix Element"=18.961370443326615}, {"Real Matrix Element"=4.095916745509522, "Real Matrix Element"=18.87129398504708}, {"Real Matrix Element"=4.238374814900775, "Real Matrix Element"=18.79016254765945}, {"Real Matrix Element"=4.122781238369786, "Real Matrix Element"=19.10914304287428}, {"Real Matrix Element"=3.9262592652126944, "Real Matrix Element"=19.112917782232074}, {"Real Matrix Element"=3.959026668394753, "Real Matrix Element"=19.182089690927977}, {"Real Matrix Element"=3.9283238031711063, "Real Matrix Element"=19.24480554799195}, {"Real Matrix Element"=3.827255286054169, "Real Matrix Element"=19.134127096792575}, {"Real Matrix Element"=3.758194149167349, "Real Matrix Element"=19.33919722686729}, {"Real Matrix Element"=3.5968381148420843, "Real Matrix Element"=19.736079596063462}, {"Real Matrix Element"=3.5265213426238917, "Real Matrix Element"=19.335581628476227}, {"Real Matrix Element"=3.339473556696922, "Real Matrix Element"=19.39958752715868}, {"Real Matrix Element"=3.322047730720935, "Real Matrix Element"=19.225281984862356}, {"Real Matrix Element"=3.2884238771143344, "Real Matrix Element"=19.38390822297435}, {"Real Matrix Element"=3.167936365146495, "Real Matrix Element"=19.31227313271643}, {"Real Matrix Element"=2.912789268579754, "Real Matrix Element"=19.303415705950957}, {"Real Matrix Element"=2.907102654450196, "Real Matrix Element"=19.43829554865164}, {"Real Matrix Element"=2.742757038156763, "Real Matrix Element"=19.681936438777278}, {"Real Matrix Element"=2.683972770487943, "Real Matrix Element"=19.56080919708144}, {"Real Matrix Element"=2.6359587788379573, "Real Matrix Element"=19.581547229758844}, {"Real Matrix Element"=2.492329588926959, "Real Matrix Element"=19.605820056538725}, {"Real Matrix Element"=2.4656499254445228, "Real Matrix Element"=19.428126533264745}, {"Real Matrix Element"=2.3633112988288305, "Real Matrix Element"=19.434639845849293}, {"Real Matrix Element"=2.2922315615513407, "Real Matrix Element"=19.834462882947143}, {"Real Matrix Element"=2.318940100045721, "Real Matrix Element"=19.56277119911333}, {"Real Matrix Element"=2.2581326973618987, "Real Matrix Element"=19.51833177124514}, {"Real Matrix Element"=2.2713210452673214, "Real Matrix Element"=20.0435820173542}, {"Real Matrix Element"=2.194464886432464, "Real Matrix Element"=19.711377530744734}, {"Real Matrix Element"=2.2922467508526623, "Real Matrix Element"=19.640158889665884}, {"Real Matrix Element"=2.2858442094114664, "Real Matrix Element"=19.635537886460526}, {"Real Matrix Element"=2.0071726300494817, "Real Matrix Element"=20.16086485269451}, {"Real Matrix Element"=1.8389647517788872, "Real Matrix Element"=20.038287113927176}, {"Real Matrix Element"=1.8020848961990863, "Real Matrix Element"=19.992704583761277}, {"Real Matrix Element"=1.7152360438707572, "Real Matrix Element"=19.943117021009833}, {"Real Matrix Element"=1.6785719675522164, "Real Matrix Element"=20.26336067770457}, {"Real Matrix Element"=1.5978842833152231, "Real Matrix Element"=20.218859923752614}, {"Real Matrix Element"=1.4690532968262648, "Real Matrix Element"=20.208213987572087}, {"Real Matrix Element"=1.3296954275537938, "Real Matrix Element"=19.98716934805409}, {"Real Matrix Element"=1.1820701654598977, "Real Matrix Element"=19.982270880457868}, {"Real Matrix Element"=1.0775449911490032, "Real Matrix Element"=19.862114555354033}, {"Real Matrix Element"=0.9210400610247974, "Real Matrix Element"=20.058365540866728}, {"Real Matrix Element"=0.8484072658179688, "Real Matrix Element"=19.92298661786653}, {"Real Matrix Element"=0.6706404018140937, "Real Matrix Element"=20.28705020172537}, {"Real Matrix Element"=0.6249168379990733, "Real Matrix Element"=20.002209519941584}, {"Real Matrix Element"=0.4744261418761635, "Real Matrix Element"=19.965498829402094}, {"Real Matrix Element"=0.39025556127631195, "Real Matrix Element"=19.97323106709498}, {"Real Matrix Element"=0.28804563293733415, "Real Matrix Element"=19.62012018820759}, {"Real Matrix Element"=0.23354009111610458, "Real Matrix Element"=19.81445128651862}, {"Real Matrix Element"=0.12976102500388786, "Real Matrix Element"=19.958473586915513}, {"Real Matrix Element"=0.08649943573329333, "Real Matrix Element"=19.780930715128235}, {"Real Matrix Element"=-0.0794017030640259, "Real Matrix Element"=19.651982974363683}, {"Real Matrix Element"=-0.22333996955272245, "Real Matrix Element"=20.33186490959596}, {"Real Matrix Element"=-0.2782082450510744, "Real Matrix Element"=20.243154351556317}, {"Real Matrix Element"=-0.294689856455728, "Real Matrix Element"=20.01250976092365}, {"Real Matrix Element"=-0.3514590931245819, "Real Matrix Element"=19.96740691580572}, {"Real Matrix Element"=-0.4559994303891428, "Real Matrix Element"=19.974708638887236}, {"Real Matrix Element"=-0.5216835882072836, "Real Matrix Element"=20.196775426219062}, {"Real Matrix Element"=-0.6283157487439895, "Real Matrix Element"=19.84994287691851}, {"Real Matrix Element"=-0.7294620068467665, "Real Matrix Element"=19.769940970122033}, {"Real Matrix Element"=-0.8303194824228229, "Real Matrix Element"=19.933595149125853}, {"Real Matrix Element"=-0.8823957652689342, "Real Matrix Element"=20.122618457965455}, {"Real Matrix Element"=-0.9843256736813639, "Real Matrix Element"=19.93845387942615}, {"Real Matrix Element"=-1.0319129569183565, "Real Matrix Element"=19.82143587420879}, {"Real Matrix Element"=-1.1627415634024372, "Real Matrix Element"=19.806326784113107}, {"Real Matrix Element"=-1.207020809393022, "Real Matrix Element"=19.782810274652803}, {"Real Matrix Element"=-1.2364425589363301, "Real Matrix Element"=19.615640090926473}, {"Real Matrix Element"=-1.311473131368317, "Real Matrix Element"=19.51394968552165}, {"Real Matrix Element"=-1.439160467034358, "Real Matrix Element"=19.48681631892193}, {"Real Matrix Element"=-1.4958513755182985, "Real Matrix Element"=19.596808799412443}, {"Real Matrix Element"=-1.5843030383880556, "Real Matrix Element"=19.69636678109708}, {"Real Matrix Element"=-1.658084464766902, "Real Matrix Element"=19.749019161250025}, {"Real Matrix Element"=-1.6511466669674546, "Real Matrix Element"=19.74066898712556}, {"Real Matrix Element"=-1.6852446862699129, "Real Matrix Element"=19.490177282960914}, {"Real Matrix Element"=-1.749579463975572, "Real Matrix Element"=19.643949717807004}, {"Real Matrix Element"=-1.8762032002195719, "Real Matrix Element"=19.673940324308937}, {"Real Matrix Element"=-1.9847941199219896, "Real Matrix Element"=19.75539004638579}, {"Real Matrix Element"=-2.0782314110873448, "Real Matrix Element"=19.606753404615745}, {"Real Matrix Element"=-2.160806674834583, "Real Matrix Element"=19.619502120290807}, {"Real Matrix Element"=-2.181584928604678, "Real Matrix Element"=19.237963210377362}, {"Real Matrix Element"=-2.2831838682738916, "Real Matrix Element"=19.17759663136179}, {"Real Matrix Element"=-2.4589126510594626, "Real Matrix Element"=19.228744137010395}, {"Real Matrix Element"=-2.4950417526789015, "Real Matrix Element"=19.39090436455205}, {"Real Matrix Element"=-2.5555108553377788, "Real Matrix Element"=19.356003455207883}, {"Real Matrix Element"=-2.690059590366169, "Real Matrix Element"=19.344273009471326}, {"Real Matrix Element"=-2.7518826840605968, "Real Matrix Element"=19.182710042891784}, {"Real Matrix Element"=-2.86810950006909, "Real Matrix Element"=19.147528934800793}, {"Real Matrix Element"=-2.9728834451333666, "Real Matrix Element"=19.241551603825588}, {"Real Matrix Element"=-3.0407590509433806, "Real Matrix Element"=19.51840762237345}, {"Real Matrix Element"=-2.9939776943623153, "Real Matrix Element"=19.248759782975412}, {"Real Matrix Element"=-3.0484994410773876, "Real Matrix Element"=19.18049632524005}, {"Real Matrix Element"=-2.960745753065656, "Real Matrix Element"=19.069094346156046}, {"Real Matrix Element"=-3.0362032170131177, "Real Matrix Element"=19.06518747915251}, {"Real Matrix Element"=-3.0799541358552958, "Real Matrix Element"=19.001419107073872}, {"Real Matrix Element"=-3.1033189651173365, "Real Matrix Element"=18.940837464777385}, {"Real Matrix Element"=-3.2115385913845045, "Real Matrix Element"=18.9622520219807}, {"Real Matrix Element"=-3.3724192143788123, "Real Matrix Element"=18.95866434198037}, {"Real Matrix Element"=-3.5213687446731545, "Real Matrix Element"=19.091479307232518}, {"Real Matrix Element"=-3.6823713655150705, "Real Matrix Element"=19.164212169531936}, {"Real Matrix Element"=-3.6069241400165017, "Real Matrix Element"=18.85457192557497}, {"Real Matrix Element"=-3.6682626331469623, "Real Matrix Element"=18.89518808817101}, {"Real Matrix Element"=-3.6695943231321535, "Real Matrix Element"=19.150472059920773}, {"Real Matrix Element"=-3.710498285169162, "Real Matrix Element"=19.03163123652101}, {"Real Matrix Element"=-3.7015016004182786, "Real Matrix Element"=18.893604451284517}, {"Real Matrix Element"=-3.63753801149407, "Real Matrix Element"=18.786690563168676}, {"Real Matrix Element"=-3.7212365785021224, "Real Matrix Element"=18.77968303347287}, {"Real Matrix Element"=-4.045183450838271, "Real Matrix Element"=18.805144052053045}, {"Real Matrix Element"=-4.004171560138177, "Real Matrix Element"=18.721002096674802}, {"Real Matrix Element"=-4.226804552960402, "Real Matrix Element"=18.85424553461262}, {"Real Matrix Element"=-4.351146834587886, "Real Matrix Element"=18.905939494788743}, {"Real Matrix Element"=-4.354021444099779, "Real Matrix Element"=19.005541570849484}, {"Real Matrix Element"=-4.555047699061901, "Real Matrix Element"=18.88697736925207}, {"Real Matrix Element"=-4.615710608935518, "Real Matrix Element"=18.834001283145543}, {"Real Matrix Element"=-4.811907876622591, "Real Matrix Element"=18.870293996016205}, {"Real Matrix Element"=-4.99150687886713, "Real Matrix Element"=18.941794186158834}, {"Real Matrix Element"=-5.184809208864786, "Real Matrix Element"=18.99326571154641}, {"Real Matrix Element"=-5.069369874097422, "Real Matrix Element"=18.86372987960499}, {"Real Matrix Element"=-5.5065449511849, "Real Matrix Element"=18.84438456070924}, {"Real Matrix Element"=-5.865352228117156, "Real Matrix Element"=18.67262039433256}, {"Real Matrix Element"=-5.881173517081438, "Real Matrix Element"=18.51829704239417}, {"Real Matrix Element"=-6.031653260894228, "Real Matrix Element"=18.35929634622047}, {"Real Matrix Element"=-6.262323771892935, "Real Matrix Element"=18.24975845542311}, {"Real Matrix Element"=-6.319043996173574, "Real Matrix Element"=18.057590471724414}, {"Real Matrix Element"=-6.320723884139767, "Real Matrix Element"=17.978553614177116}, {"Real Matrix Element"=-6.537001936365448, "Real Matrix Element"=17.95365674456965}, {"Real Matrix Element"=-6.425602227657636, "Real Matrix Element"=17.688454207241207}, {"Real Matrix Element"=-6.323539911176449, "Real Matrix Element"=17.521195299298313}, {"Real Matrix Element"=-6.3501474529869615, "Real Matrix Element"=17.461473691599664}, {"Real Matrix Element"=-6.224792556214783, "Real Matrix Element"=17.227025057761082}, {"Real Matrix Element"=-6.4633243133131755, "Real Matrix Element"=17.287556849713116}, {"Real Matrix Element"=-6.6061241520755924, "Real Matrix Element"=17.251722118906944}, {"Real Matrix Element"=-6.616941515492813, "Real Matrix Element"=17.17516771870752}, {"Real Matrix Element"=-6.699444991640118, "Real Matrix Element"=17.11044998609083}, {"Real Matrix Element"=-6.637195526184825, "Real Matrix Element"=16.94588425513183}, {"Real Matrix Element"=-6.598680039269585, "Real Matrix Element"=16.99572273445465}, {"Real Matrix Element"=-6.5815219595206615, "Real Matrix Element"=16.884656861506915}, {"Real Matrix Element"=-6.766573572433235, "Real Matrix Element"=17.019517265179356}, {"Real Matrix Element"=-6.5913156580244765, "Real Matrix Element"=16.81039472224616}, {"Real Matrix Element"=-6.631109175631318, "Real Matrix Element"=16.764706100757518}, {"Real Matrix Element"=-6.697556603011058, "Real Matrix Element"=16.763983871240814}, {"Real Matrix Element"=-6.707361691013661, "Real Matrix Element"=16.7117627504171}, {"Real Matrix Element"=-6.658886576075322, "Real Matrix Element"=16.599813418514675}, {"Real Matrix Element"=-6.99949876260425, "Real Matrix Element"=16.60252027035554}, {"Real Matrix Element"=-7.108404430136151, "Real Matrix Element"=16.233162544838454}, {"Real Matrix Element"=-7.016660980584992, "Real Matrix Element"=15.786615254842621}, {"Real Matrix Element"=-7.163915696198325, "Real Matrix Element"=15.875791028916408}, {"Real Matrix Element"=-7.200415150551832, "Real Matrix Element"=15.69359364983884}, {"Real Matrix Element"=-7.305663984822154, "Real Matrix Element"=15.616995822683249}, {"Real Matrix Element"=-7.350419958532535, "Real Matrix Element"=15.720408711619855}, {"Real Matrix Element"=-7.341909899051574, "Real Matrix Element"=15.574152209327302}, {"Real Matrix Element"=-7.30471426001636, "Real Matrix Element"=15.351616409902105}, {"Real Matrix Element"=-7.270503730787275, "Real Matrix Element"=15.271941426351653}, {"Real Matrix Element"=-7.284160382818166, "Real Matrix Element"=15.299457232674865}, {"Real Matrix Element"=-7.433573509313121, "Real Matrix Element"=15.336503390635674}, {"Real Matrix Element"=-7.476391789600023, "Real Matrix Element"=15.38441342233676}, {"Real Matrix Element"=-7.628555167223143, "Real Matrix Element"=15.282243963958624}, {"Real Matrix Element"=-7.424914255864464, "Real Matrix Element"=14.911053738930754}, {"Real Matrix Element"=-7.504187224729142, "Real Matrix Element"=14.550879236933538}, {"Real Matrix Element"=-7.533558391457788, "Real Matrix Element"=14.677131552374439}, {"Real Matrix Element"=-7.587724338411188, "Real Matrix Element"=14.46445161276539}, {"Real Matrix Element"=-7.608433231751784, "Real Matrix Element"=14.635682956859313}, {"Real Matrix Element"=-7.711901184049588, "Real Matrix Element"=14.75985149669739}, {"Real Matrix Element"=-7.709987965475114, "Real Matrix Element"=14.524182128292347}, {"Real Matrix Element"=-7.789944504052315, "Real Matrix Element"=14.358061000458926}, {"Real Matrix Element"=-8.022225957329143, "Real Matrix Element"=14.421504010991214}, {"Real Matrix Element"=-8.161633625968204, "Real Matrix Element"=14.232455086905244}, {"Real Matrix Element"=-8.120141149384924, "Real Matrix Element"=14.21273614584257}, {"Real Matrix Element"=-8.292914654417483, "Real Matrix Element"=14.412109588687088}, {"Real Matrix Element"=-8.33580136705327, "Real Matrix Element"=14.186776461096027}, {"Real Matrix Element"=-8.319497855807507, "Real Matrix Element"=14.07489296864824}, {"Real Matrix Element"=-8.266752625074249, "Real Matrix Element"=14.116527203636423}, {"Real Matrix Element"=-8.226447872869958, "Real Matrix Element"=14.014632012876397}, {"Real Matrix Element"=-8.266194595569896, "Real Matrix Element"=13.802955413031784}, {"Real Matrix Element"=-8.46136067981557, "Real Matrix Element"=13.849562322269366}, {"Real Matrix Element"=-8.475847103440447, "Real Matrix Element"=13.915222127082302}, {"Real Matrix Element"=-8.365312108979728, "Real Matrix Element"=13.658325360225541}, {"Real Matrix Element"=-8.47227038572879, "Real Matrix Element"=13.577319154808634}, {"Real Matrix Element"=-8.599492111084832, "Real Matrix Element"=13.421644686324187}, {"Real Matrix Element"=-8.615401903342514, "Real Matrix Element"=13.355062791269404}, {"Real Matrix Element"=-8.613128016559488, "Real Matrix Element"=13.310475747001338}, {"Real Matrix Element"=-8.563789834170931, "Real Matrix Element"=13.140458454885872}, {"Real Matrix Element"=-8.607921556052654, "Real Matrix Element"=12.990700070489607}, {"Real Matrix Element"=-8.589670203171867, "Real Matrix Element"=12.868980047849087}, {"Real Matrix Element"=-8.553927533316642, "Real Matrix Element"=12.735293289858266}, {"Real Matrix Element"=-8.697829768728088, "Real Matrix Element"=12.737620135460585}, {"Real Matrix Element"=-8.765182015259311, "Real Matrix Element"=12.524850442435042}, {"Real Matrix Element"=-8.6838398372976, "Real Matrix Element"=12.502717195847525}, {"Real Matrix Element"=-8.671888624729513, "Real Matrix Element"=12.434090320507124}, {"Real Matrix Element"=-8.66493119697179, "Real Matrix Element"=12.363677726291451}, {"Real Matrix Element"=-8.582458701623445, "Real Matrix Element"=12.398426682260249}, {"Real Matrix Element"=-8.502637959780627, "Real Matrix Element"=12.297045715032377}, {"Real Matrix Element"=-8.594585797941468, "Real Matrix Element"=12.266590177774557}, {"Real Matrix Element"=-8.523078958748012, "Real Matrix Element"=11.981773222023051}, {"Real Matrix Element"=-8.608517194392284, "Real Matrix Element"=11.935961130852094}, {"Real Matrix Element"=-8.657425308154185, "Real Matrix Element"=11.77737175443987}, {"Real Matrix Element"=-8.62916071069874, "Real Matrix Element"=11.423529719395248}, {"Real Matrix Element"=-8.770797293061408, "Real Matrix Element"=11.425350016572407}, {"Real Matrix Element"=-8.806619074685075, "Real Matrix Element"=11.562753979402162}, {"Real Matrix Element"=-8.545119820976291, "Real Matrix Element"=11.234646944753692}, {"Real Matrix Element"=-8.758852861401616, "Real Matrix Element"=11.327505749849914}, {"Real Matrix Element"=-8.607594446567203, "Real Matrix Element"=11.172264709871957}, {"Real Matrix Element"=-8.596517930059285, "Real Matrix Element"=10.985780549364987}, {"Real Matrix Element"=-8.67176691248744, "Real Matrix Element"=10.813571076941189}, {"Real Matrix Element"=-8.895090333924198, "Real Matrix Element"=10.701626935162926}, {"Real Matrix Element"=-8.696172692211519, "Real Matrix Element"=10.475042957185867}, {"Real Matrix Element"=-8.73291818646375, "Real Matrix Element"=10.53081545885271}, {"Real Matrix Element"=-8.61016060689553, "Real Matrix Element"=10.359062360186455}, {"Real Matrix Element"=-8.752347130697242, "Real Matrix Element"=10.275768450255256}, {"Real Matrix Element"=-8.876469268973743, "Real Matrix Element"=10.336037357356068}, {"Real Matrix Element"=-8.661091922455329, "Real Matrix Element"=10.027554334047968}, {"Real Matrix Element"=-8.821125238461073, "Real Matrix Element"=9.950406193420655}, {"Real Matrix Element"=-8.900035600989638, "Real Matrix Element"=9.774072940368846}, {"Real Matrix Element"=-8.93742722541149, "Real Matrix Element"=9.955614845814228}, {"Real Matrix Element"=-8.852700322466326, "Real Matrix Element"=9.572881051224366}, {"Real Matrix Element"=-8.843104588170531, "Real Matrix Element"=9.294720573613299}, {"Real Matrix Element"=-8.806639011877134, "Real Matrix Element"=8.9703686415516}, {"Real Matrix Element"=-8.758586939542665, "Real Matrix Element"=9.058896327978724}, {"Real Matrix Element"=-8.737768179536632, "Real Matrix Element"=8.947668624641432}, {"Real Matrix Element"=-8.641513281085606, "Real Matrix Element"=8.984584043551187}, {"Real Matrix Element"=-8.544756198689061, "Real Matrix Element"=8.837774962974086}, {"Real Matrix Element"=-8.607163812819874, "Real Matrix Element"=8.716542665080173}, {"Real Matrix Element"=-8.621300258703268, "Real Matrix Element"=8.560862410756734}, {"Real Matrix Element"=-8.69901681867739, "Real Matrix Element"=8.547709427608108}, {"Real Matrix Element"=-8.873995689698644, "Real Matrix Element"=8.714745884590187}, {"Real Matrix Element"=-9.012488263663153, "Real Matrix Element"=8.68522647591172}, {"Real Matrix Element"=-8.90594304455854, "Real Matrix Element"=8.335778858666083}, {"Real Matrix Element"=-8.961134050741647, "Real Matrix Element"=8.325291473174563}, {"Real Matrix Element"=-8.835293927253971, "Real Matrix Element"=7.884463934491831}, {"Real Matrix Element"=-9.064804645573721, "Real Matrix Element"=7.998676123983236}, {"Real Matrix Element"=-9.22305446878618, "Real Matrix Element"=7.92064043990446}, {"Real Matrix Element"=-9.06603806339783, "Real Matrix Element"=7.525179596824946}, {"Real Matrix Element"=-9.089733580702894, "Real Matrix Element"=7.566400016850758}, {"Real Matrix Element"=-9.018487210784922, "Real Matrix Element"=7.4424344445384545}, {"Real Matrix Element"=-8.9890242487483, "Real Matrix Element"=7.247930974899337}, {"Real Matrix Element"=-8.980328261757354, "Real Matrix Element"=7.171983513315269}, {"Real Matrix Element"=-8.917248372735617, "Real Matrix Element"=7.204351667849104}, {"Real Matrix Element"=-8.828461783924805, "Real Matrix Element"=7.045654401750913}, {"Real Matrix Element"=-8.729588618619033, "Real Matrix Element"=6.9907506579676175}, {"Real Matrix Element"=-8.580447519996067, "Real Matrix Element"=6.877767424499953}, {"Real Matrix Element"=-8.534791173015968, "Real Matrix Element"=6.697714297148076}, {"Real Matrix Element"=-8.602355275725017, "Real Matrix Element"=6.752442544481637}, {"Real Matrix Element"=-8.519045154756789, "Real Matrix Element"=6.584126973226976}, {"Real Matrix Element"=-8.509785443864327, "Real Matrix Element"=6.653634355935767}, {"Real Matrix Element"=-8.579038119396245, "Real Matrix Element"=6.649409382224908}, {"Real Matrix Element"=-8.611332795782301, "Real Matrix Element"=6.764279288769613}, {"Real Matrix Element"=-8.425657255125557, "Real Matrix Element"=6.556596117251381}, {"Real Matrix Element"=-8.235986868760735, "Real Matrix Element"=6.414497073863071}, {"Real Matrix Element"=-8.181692306943606, "Real Matrix Element"=6.286713563077992}, {"Real Matrix Element"=-8.136947416464052, "Real Matrix Element"=6.329023819071581}, {"Real Matrix Element"=-8.143848597314673, "Real Matrix Element"=6.359499744559379}, {"Real Matrix Element"=-8.055279858231813, "Real Matrix Element"=6.134251739985477}, {"Real Matrix Element"=-8.0700826610748, "Real Matrix Element"=6.176475378197828}, {"Real Matrix Element"=-8.222131574591224, "Real Matrix Element"=6.187350393054747}, {"Real Matrix Element"=-8.286357577330683, "Real Matrix Element"=6.118247537301858}, {"Real Matrix Element"=-8.114445945755929, "Real Matrix Element"=6.030932407744156}, {"Real Matrix Element"=-8.210074215141848, "Real Matrix Element"=5.979004791113523}, {"Real Matrix Element"=-8.312680087244612, "Real Matrix Element"=5.868629668722855}, {"Real Matrix Element"=-8.404227732532323, "Real Matrix Element"=5.730448389287154}, {"Real Matrix Element"=-8.118015049175295, "Real Matrix Element"=5.581906978966135}, {"Real Matrix Element"=-8.043499519030737, "Real Matrix Element"=5.44685304823719}, {"Real Matrix Element"=-7.930604543363039, "Real Matrix Element"=5.284349804771601}, {"Real Matrix Element"=-7.685490700884913, "Real Matrix Element"=5.113562755387711}, {"Real Matrix Element"=-7.746469212369693, "Real Matrix Element"=5.087559413259944}, {"Real Matrix Element"=-7.694412202370247, "Real Matrix Element"=4.895973884573735}, {"Real Matrix Element"=-7.662726197640507, "Real Matrix Element"=4.771690442716227}, {"Real Matrix Element"=-7.72554952119642, "Real Matrix Element"=4.584302922812276}, {"Real Matrix Element"=-7.833164032945452, "Real Matrix Element"=4.477523870291501}, {"Real Matrix Element"=-7.870671296950889, "Real Matrix Element"=4.375271456970237}, {"Real Matrix Element"=-7.699187192309577, "Real Matrix Element"=4.206567644074009}, {"Real Matrix Element"=-7.6350744100441865, "Real Matrix Element"=3.9873549691380985}, {"Real Matrix Element"=-7.552848395090781, "Real Matrix Element"=3.932400498920551}, {"Real Matrix Element"=-7.425343562187817, "Real Matrix Element"=3.7705200104985757}, {"Real Matrix Element"=-7.338341439370567, "Real Matrix Element"=3.908283898961539}, {"Real Matrix Element"=-7.319673469461896, "Real Matrix Element"=4.021787319154243}, {"Real Matrix Element"=-7.287938346655437, "Real Matrix Element"=3.9054834192648538}, {"Real Matrix Element"=-7.218306177241856, "Real Matrix Element"=3.8748066018247096}, {"Real Matrix Element"=-7.27656941071718, "Real Matrix Element"=3.831279586331392}, {"Real Matrix Element"=-7.197903496336639, "Real Matrix Element"=3.5271526350503626}, {"Real Matrix Element"=-7.2383762233943445, "Real Matrix Element"=3.3338346841605966}, {"Real Matrix Element"=-7.093776469290139, "Real Matrix Element"=3.3314518445135493}, {"Real Matrix Element"=-7.097100027925128, "Real Matrix Element"=3.4347098479350215}, {"Real Matrix Element"=-6.8343309526871, "Real Matrix Element"=3.3898982020396335}, {"Real Matrix Element"=-6.7171142099878685, "Real Matrix Element"=3.2028518217559623}, {"Real Matrix Element"=-6.74473487964619, "Real Matrix Element"=3.1428087024193863}, {"Real Matrix Element"=-6.439143638067814, "Real Matrix Element"=2.9933366625530207}, {"Real Matrix Element"=-6.432000315186142, "Real Matrix Element"=2.9173481726375217}, {"Real Matrix Element"=-6.396895662309998, "Real Matrix Element"=3.020869288022181}, {"Real Matrix Element"=-6.271029351030735, "Real Matrix Element"=2.955077255505709}, {"Real Matrix Element"=-6.094647330906733, "Real Matrix Element"=2.842463919594082}, {"Real Matrix Element"=-6.019835764811554, "Real Matrix Element"=2.800947523983382}, {"Real Matrix Element"=-5.922034402021082, "Real Matrix Element"=2.9217009420504265}, {"Real Matrix Element"=-5.751343373970012, "Real Matrix Element"=2.699519424098439}, {"Real Matrix Element"=-5.633429962189656, "Real Matrix Element"=2.659861152288904}, {"Real Matrix Element"=-5.6519733511137265, "Real Matrix Element"=2.4954527961600297}, {"Real Matrix Element"=-5.5879146859871245, "Real Matrix Element"=2.3508932582900828}, {"Real Matrix Element"=-5.506346677869171, "Real Matrix Element"=2.2134979148399627}, {"Real Matrix Element"=-5.501111242134763, "Real Matrix Element"=2.348765950485406}, {"Real Matrix Element"=-5.4942258815609035, "Real Matrix Element"=2.3934512716345027}, {"Real Matrix Element"=-5.531927097521007, "Real Matrix Element"=2.2426566073809573}, {"Real Matrix Element"=-5.6510446376105445, "Real Matrix Element"=2.2777390025227153}, {"Real Matrix Element"=-5.531352701848458, "Real Matrix Element"=2.3598120983814086}, {"Real Matrix Element"=-5.432169037530528, "Real Matrix Element"=2.2407897452078456}, {"Real Matrix Element"=-5.371536701946831, "Real Matrix Element"=2.2270687968214045}, {"Real Matrix Element"=-5.406607040795495, "Real Matrix Element"=2.1367167370925997}, {"Real Matrix Element"=-5.288511873962015, "Real Matrix Element"=2.075338066482354}, {"Real Matrix Element"=-5.193809611594917, "Real Matrix Element"=2.06113795512699}, {"Real Matrix Element"=-5.069119135676416, "Real Matrix Element"=1.9925176847042287}, {"Real Matrix Element"=-4.893610213995878, "Real Matrix Element"=1.91219382972363}, {"Real Matrix Element"=-4.815458337428809, "Real Matrix Element"=2.022346653444013}, {"Real Matrix Element"=-4.797937963815076, "Real Matrix Element"=2.0163640913854484}, {"Real Matrix Element"=-4.7775651897131315, "Real Matrix Element"=1.8649434520237238}, {"Real Matrix Element"=-4.5013594467833205, "Real Matrix Element"=1.6528474224697818}, {"Real Matrix Element"=-4.441309890737685, "Real Matrix Element"=1.5192816964026215}, {"Real Matrix Element"=-4.2281973839104, "Real Matrix Element"=1.4416446000658716}, {"Real Matrix Element"=-4.365208412728094, "Real Matrix Element"=1.4041089455549467}, {"Real Matrix Element"=-4.13667750398369, "Real Matrix Element"=1.234124732196859}, {"Real Matrix Element"=-4.040035048127384, "Real Matrix Element"=1.1420054271397981}, {"Real Matrix Element"=-3.891678650817078, "Real Matrix Element"=0.9697658877670714}, {"Real Matrix Element"=-3.9372192232738006, "Real Matrix Element"=1.1084182327600092}, {"Real Matrix Element"=-3.899651992137444, "Real Matrix Element"=1.1725933183732697}, {"Real Matrix Element"=-3.7479010357596643, "Real Matrix Element"=1.086527061253903}, {"Real Matrix Element"=-3.705236859000565, "Real Matrix Element"=0.8887407341569953}, {"Real Matrix Element"=-3.5493485074104854, "Real Matrix Element"=0.6143951929270575}, {"Real Matrix Element"=-3.5709904016765575, "Real Matrix Element"=0.5794481074182778}, {"Real Matrix Element"=-3.533253910557299, "Real Matrix Element"=0.4681155643051908}, {"Real Matrix Element"=-3.3938826328746696, "Real Matrix Element"=0.3831987842455438}, {"Real Matrix Element"=-3.2468143357879375, "Real Matrix Element"=0.3275826052600016}, {"Real Matrix Element"=-3.232536395502047, "Real Matrix Element"=0.3941107361964644}, {"Real Matrix Element"=-3.0870171060031124, "Real Matrix Element"=0.6744201265766647}, {"Real Matrix Element"=-2.9009884258715184, "Real Matrix Element"=0.48179929339738137}, {"Real Matrix Element"=-2.6850723741981595, "Real Matrix Element"=0.4505541772689051}, {"Real Matrix Element"=-2.366756991137511, "Real Matrix Element"=0.4045770314889004}, {"Real Matrix Element"=-2.4163183293779, "Real Matrix Element"=0.6447279111490565}, {"Real Matrix Element"=-2.4386672243412786, "Real Matrix Element"=0.5971958903355987}, {"Real Matrix Element"=-2.46255893660953, "Real Matrix Element"=0.5216491790100619}, {"Real Matrix Element"=-2.4473974549145434, "Real Matrix Element"=0.4483995844576454}, {"Real Matrix Element"=-2.229510967931882, "Real Matrix Element"=0.32178991165044096}, {"Real Matrix Element"=-2.24527108102615, "Real Matrix Element"=0.2647607192645737}, {"Real Matrix Element"=-2.239731890354996, "Real Matrix Element"=0.3501550741786431}, {"Real Matrix Element"=-2.163894139051156, "Real Matrix Element"=0.41263961211096223}, {"Real Matrix Element"=-2.087372780379963, "Real Matrix Element"=0.2627963576119685}, {"Real Matrix Element"=-1.9311455819719665, "Real Matrix Element"=0.23057274833627456}, {"Real Matrix Element"=-1.7390382574008312, "Real Matrix Element"=0.08229283641021495}, {"Real Matrix Element"=-1.6454627299896398, "Real Matrix Element"=0.13753015484421}, {"Real Matrix Element"=-1.5521898865492718, "Real Matrix Element"=0.26147720281785536}, {"Real Matrix Element"=-1.4271137533562612, "Real Matrix Element"=0.20800753627190915}]}, ...(3 in all)]
  in  "DT":dbl=0.1
  out "time":dbl
  in  "정지":bool
  in  "y variance":dbl=0.1
  in  "x variance":dbl=0.1
  in  "observation y covariance":dbl=1.0
  in  "observation x covariance":dbl=1.0
  in  "gps y covariance":dbl=0.5
  in  "gps x covariance":dbl=0.5
  in  "noise deg":dbl=30.0
  in  "noise len":dbl=1.0
  in  "yaw variance":dbl=1.0 format="%#_13g"
  in  "vel variance":dbl=1.0 format="%#_13g"
  # "Extended Kalman Filter"
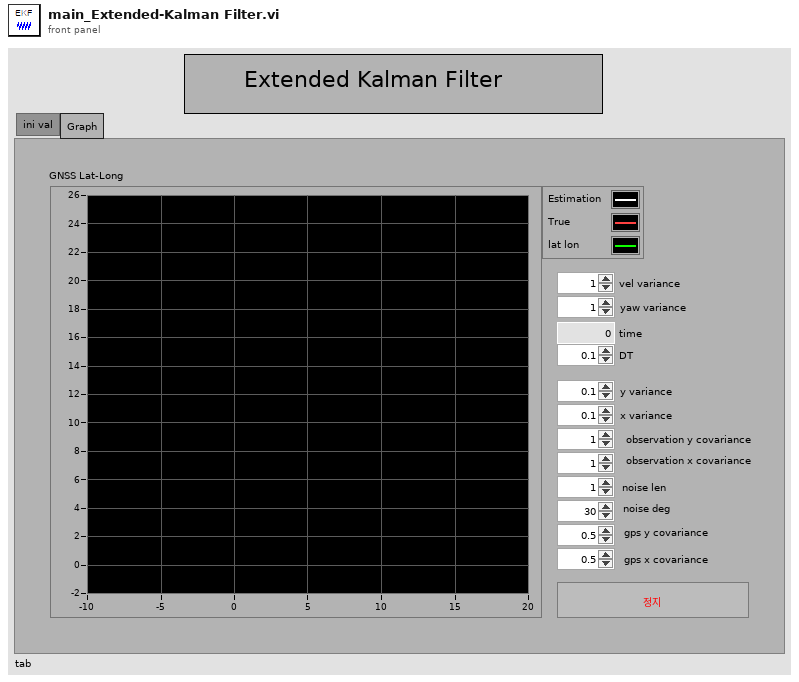
[diagram p1: front panel]
types:
  T1 = cluster{cluster{"Real Matrix Element":dbl, "Real Matrix Element":dbl}[]}[]
  T2 = typedef "cmd_common.ctl" = enum16{"read", "write"}
  T3 = typedef "cmd_ini-RW.ctl" = enum16{"ini", "read", "write"}
  T4 = typedef "NI_Matrix.lvlib/RealMatrix.ctl" = dbl[][]
  T5 = cluster{"Real Matrix":T4, "Real Matrix":T4, "Real Matrix":T4, "Real Matrix":T4, "Real Matrix":T4}
  T6 = cluster{"xEst":T4, "xTrue":T4, "PEst":T4, "xDR":T4, "hz":T4}
  T7 = cluster{"Real Matrix Element":dbl, "Real Matrix Element":dbl}
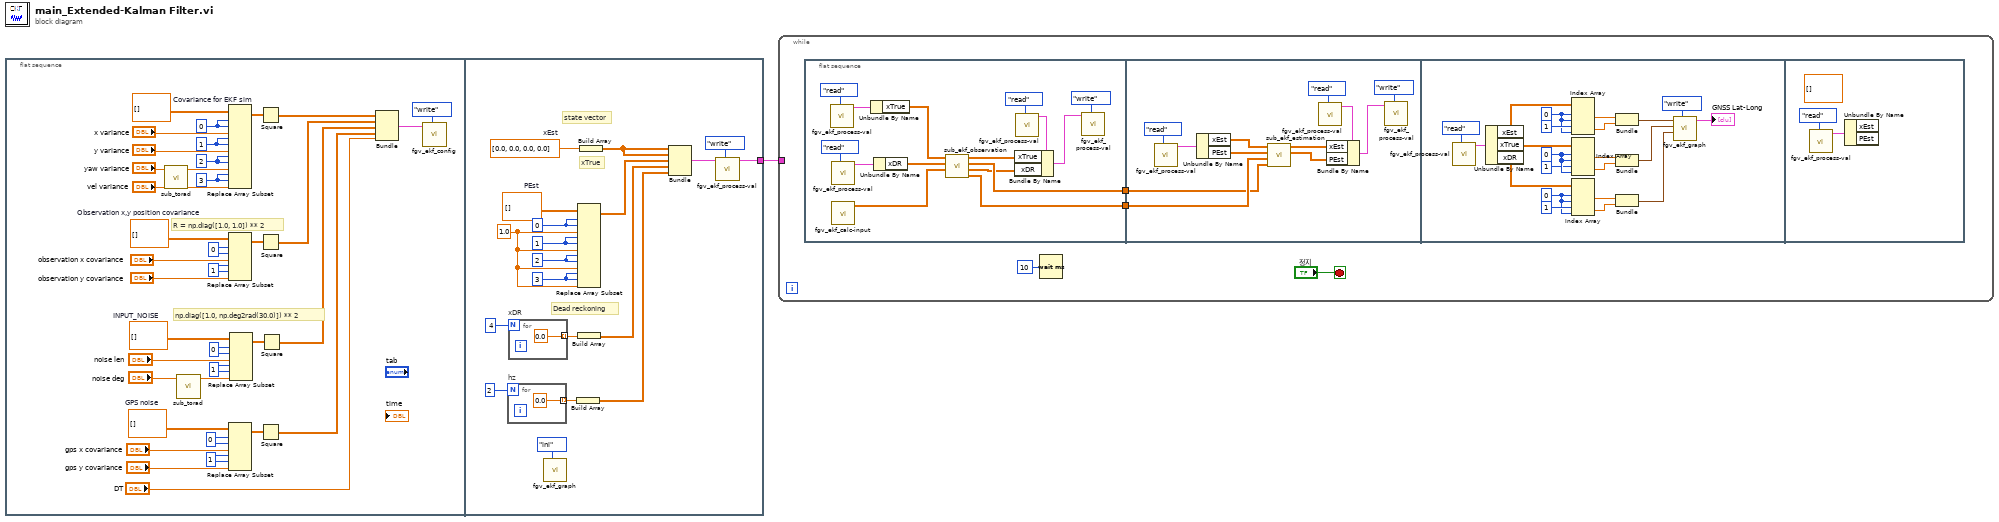
[diagram p0: block diagram]
diagram:
  n1 = flat-sequence {
    tunnel: [w40] -> w1
    frame #0 {
      w11 = 1 ("index (row)")
      w12 = 0 ("disabled index (row)")
      w8 = T4 []  # INPUT_NOISE
      w14 = 3 ("index (row)")
      w17 = 1 ("index (row)")
      w16 = 0 ("disabled index (row)")
      w21 = T4 []  # GPS noise
      w27 = 1 ("index (row)")
      w28 = 0 ("disabled index (row)")
      w23 = T4 []  # Observation x,y position covariance
      w30 = 2 ("index (row)")
      w37 = 1 ("index (row)")
      w38 = 0 ("disabled index (row)")
      w33 = T4 []  # Covariance for EKF sim
      # "np.diag([1.0, np.deg2rad(30.0)]) ** 2"
      # "R = np.diag([1.0, 1.0]) ** 2"
      n2 = call "sub_torad.vi"("φ"="yaw variance") -> ("rad"=w31:dbl)  [unwired: 10 in]
      n3 = call "sub_torad.vi"("φ"="noise deg") -> ("rad"=w3:dbl)  [unwired: 10 in]
      n4 = Replace Array Subset(array=w33, new element #1="x variance", index (row) #1=w38, index (col) #1=w38, new element #2="y variance", index (row) #2=w37, index (col) #2=w37, new element #3=w31, index (row) #3=w30, index (col) #3=w30, new element #4="vel variance", index (row) #4=w14, index (col) #4=w14) -> (w36:T4)
      n5 = Replace Array Subset(array=w23, new element #1="observation x covariance", index (row) #1=w28, index (col) #1=w28, new element #2="observation y covariance", index (row) #2=w27, index (col) #2=w27) -> (w26:T4)
      n6 = Replace Array Subset(array=w21, new element #1="gps x covariance", index (row) #1=w16, index (col) #1=w16, new element #2="gps y covariance", index (row) #2=w17, index (col) #2=w17) -> (w18:T4)
      n7 = Replace Array Subset(array=w8, new element #1="noise len", index (row) #1=w12, index (col) #1=w12, new element #2=w3, index (row) #2=w11, index (col) #2=w11) -> (w10:T4)
      n8 = Square(x=w36) -> (x^2=w29:T4)
      n9 = Square(x=w26) -> (x^2=w22:T4)
      n10 = Square(x=w18) -> (x^2=w15:T4)
      n11 = Square(x=w10) -> (x^2=w7:T4)
      n12 = Bundle(w29, w22, w7, w15, "DT"="DT") -> (w6:cluster{T4, T4, T4, T4, "DT":dbl})  [unwired: 1 in]
      n13 = call "fgv_ekf_config.vi"("cmd"=cmd_common."write", "set var"=w6) -> ()  [unwired: 9 in, 1 out]
    }
    frame #1 {
      w49 = 1.0 ("new diagonal/fill element")
      w50 = 3 ("index (row)")
      w51 = 2 ("index (row)")
      w53 = 1 ("index (row)")
      w54 = 0 ("disabled index (row)")
      w52 = T4 []  # PEst
      w55 = dbl[] [0.0, 0.0, 0.0, 0.0]  # xEst
      # "xTrue"
      # "Dead reckoning"
      # "state vector"
      n14 = for "hz" {
        N: 2 -> [_]
        tunnel: [0.0] -> w44 mode=indexing
      }
      n15 = for "xDR" {
        N: 4 -> [_]
        tunnel: [0.0] -> w57 mode=indexing
      }
      n16 = call "fgv_ekf_graph.vi"("cmd"=cmd_ini-RW."ini") -> ()  [unwired: 10 in, 1 out]
      n17 = Build Array(w44) -> (w43:T4)
      n18 = Replace Array Subset(array=w52, new element #1=w49, index (row) #1=w54, index (col) #1=w54, new element #2=w49, index (row) #2=w53, index (col) #2=w53, new element #3=w49, index (row) #3=w51, index (col) #3=w51, new element #4=w49, index (row) #4=w50, index (col) #4=w50) -> (w47:T4)
      n19 = Build Array(w57) -> (w46:T4)
      n20 = Build Array(w55) -> (w48:T4)
      n21 = Bundle("Real Matrix"=w48, "Real Matrix"=w48, "Real Matrix"=w47, "Real Matrix"=w46, "Real Matrix"=w43) -> (w42:T5)  [unwired: 1 in]
      n22 = call "fgv_ekf_process-val.vi"("cmd"=cmd_common."write", "process val"=w42) -> ("process val out"=w40:T6)  [unwired: 9 in]
    }
  }
  n23 = while {
    tunnel: w1 -> [_]
    stop <- "정지" stop-if-true
    n24 = flat-sequence {
      tunnel: [w78] -> w62
      tunnel: [w77] -> w61
      tunnel: w62 -> [w86]
      tunnel: w61 -> [w88]
      frame #0 {
        n25 = call "fgv_ekf_process-val.vi"("cmd"=cmd_common."read") -> ("process val out"=w67:T6)  [unwired: 10 in]
        n26 = call "fgv_ekf_process-val.vi"("cmd"=cmd_common."read") -> ("process val out"=w65:T6)  [unwired: 10 in]
        n27 = call "fgv_ekf_calc-input.vi"() -> ("u"=w70:T4)  [unwired: 11 in]
        n28 = Unbundle By Name(w67) -> ("xTrue"=w69:T4)
        n29 = Unbundle By Name(w65) -> ("xDR"=w68:T4)
        n30 = call "sub_ekf_observation.vi"("u"=w70, "xDR"=w68, "xTrue"=w69) -> ("ud"=w77:T4, "xDR"=w72:T4, "z"=w78:T4, "x_true out"=w73:T4)  [unwired: 5 in]
        n31 = call "fgv_ekf_process-val.vi"("cmd"=cmd_common."read") -> ("process val out"=w75:T6)  [unwired: 10 in]
        n32 = Bundle By Name(cluster=w75, "xTrue"=w73, "xDR"=w72) -> (w76:T6)
        n33 = call "fgv_ekf_process-val.vi"("cmd"=cmd_common."write", "process val"=w76) -> ()  [unwired: 9 in, 1 out]
      }
      frame #1 {
        n34 = call "fgv_ekf_process-val.vi"("cmd"=cmd_common."read") -> ("process val out"=w89:T6)  [unwired: 10 in]
        n35 = Unbundle By Name(w89) -> ("xEst"=w85:T4, "PEst"=w87:T4)
        n36 = call "sub_ekf_estimation.vi"("z"=w86, "ud"=w88, "PEst"=w87, "xEst"=w85) -> ("PEst"=w79:T4, "xEst"=w81:T4)  [unwired: 6 in]
        n37 = call "fgv_ekf_process-val.vi"("cmd"=cmd_common."read") -> ("process val out"=w83:T6)  [unwired: 10 in]
        n38 = Bundle By Name(cluster=w83, "xEst"=w81, "PEst"=w79) -> (w82:T6)
        n39 = call "fgv_ekf_process-val.vi"("cmd"=cmd_common."write", "process val"=w82) -> ()  [unwired: 9 in, 1 out]
      }
      frame #2 {
        w99 = 0 ("index (row)")
        w106 = 0 ("index (row)")
        w107 = 0 ("index (row)")
        n40 = call "fgv_ekf_process-val.vi"("cmd"=cmd_common."read") -> ("process val out"=w97:T6)  [unwired: 10 in]
        n41 = Unbundle By Name(w97) -> ("xEst"=w96:T4, "xTrue"=w95:T4, "xDR"=w94:T4)
        n42 = Index Array(array=w96, index (row) #1=w107, index (col) #1=w107, index (row) #2=1 ("index (row)"), index (col) #2=w107) -> (element #1=w109:dbl, element #2=w110:dbl)
        n43 = Index Array(array=w95, index (row) #1=w106, index (col) #1=w106, index (row) #2=1 ("index (row)"), index (col) #2=w106) -> (element #1=w104:dbl, element #2=w103:dbl)
        n44 = Index Array(array=w94, index (row) #1=w99, index (col) #1=w99, index (row) #2=1 ("index (row)"), index (col) #2=w99) -> (element #1=w101:dbl, element #2=w102:dbl)
        n45 = Bundle("Real Matrix Element"=w109, "Real Matrix Element"=w110) -> (w93:T7)  [unwired: 1 in]
        n46 = Bundle("Real Matrix Element"=w104, "Real Matrix Element"=w103) -> (w92:T7)  [unwired: 1 in]
        n47 = Bundle("Real Matrix Element"=w101, "Real Matrix Element"=w102) -> (w91:T7)  [unwired: 1 in]
        n48 = call "fgv_ekf_graph.vi"("cmd"=cmd_ini-RW."write", "x_dr"=w91, "x_true"=w92, "x_est"=w93) -> ("Graph sum"=→"GNSS Lat-Long":cluster{cluster{"x":dbl, "y":dbl}[]}[])  [unwired: 7 in]
      }
      frame #3 {
        (unwired) T4 [] ("xEst")
        n49 = call "fgv_ekf_process-val.vi"("cmd"=cmd_common."read") -> ("process val out"=w114:T6)  [unwired: 10 in]
        n50 = Unbundle By Name(w114) -> ()  [unwired: 2 out]
      }
    }
    n51 = Wait (ms)(milliseconds to wait=u32 10 ("대기 시간 (ms)")) -> ()  [unwired: 1 out]
  }
